vi "Autonomous Independent.vi"   [LabVIEW 2014]
doc: "This VI is called when autonomous begins, and will automatically be terminated when autonomous ends. You can carry out timed or sensor driven robot movement independently without needing to return to the caller."
uses:
  <vilib>/Rock Robotics/WPI/Relay/WPI_RelayValue.ctl
  <vilib>/Rock Robotics/Network Tables/SD Read String.vi
  <vilib>/Rock Robotics/WPI/RobotDrive/WPI_RobotDriveGetSetRefNum.vi
  Robot Global Data.vi
  <vilib>/Rock Robotics/WPI/RobotDrive/WPI_RobotDriveMecanumDrive_Cartesian.vi
  <vilib>/addons/control/pid/pid.llb/PID (DBL).vi
  <vilib>/Rock Robotics/Network Tables/SD Write Number.vi
  <vilib>/Rock Robotics/Network Tables/SD Write Numeric Array.vi
  SimpleGyro/SimpleGyro.lvlib
  <vilib>/addons/control/pid/NI_PID_pid.lvlib
panel:
  # "Be sure to right-click and choose Data Operations>>Make Current Value default if you want to save the array values with the VI"
types:
  T1 = typedef "WPI_RelayValue.ctl" = enum16{"Off", "On", "Forward", "Reverse"}
  T2 = cluster{"proportional gain (Kc)":dbl, "integral time (Ti, min)":dbl, "derivative time (Td, min)":dbl}
  T3 = typedef "SimpleGyro.lvlib/WPI_SimpleGyroDevRef.ctl" = cluster{"DevStatus":errorcluster, "Handle":i32, "Controller":T4, "SPI Bus":T5, "Device Found":bool, "Sample Rate":dbl}
  T4 = typedef "FPGA_TypedefDigitalModule.ctl" = enum16{"Controller 1"}
  T5 = typedef "spi_bus.ctl" = enum16{"SPI On-Board, CS0", "SPI On-Board, CS1", "SPI On-Board, CS2", "SPI On-Board, CS3", "SPI MXP", "Invalid"}
  T6 = typedef "WPI_RobotDriveDevRef.ctl" = cluster{"DevStatus":errorcluster, "Motors[]":T7[], "Square Inputs":bool, "Max Output":dbl}
  T7 = typedef "WPI_MotorControlDeviceRef.ctl" = cluster{"DeviceStatus":errorcluster, "Type":T8, "PWM":cluster{"Controller":T4, "PWM Channel":T9, "DeadBand":T10}, "CAN":cluster{"Device Number":u8, "Control Mode":T11, "Semaphore":T12, "Max Vout":dbl, "TalonSRX Control Mode":T13}, "Invert":bool, "TransformRef":T14, "InvTransformRef":T14}
  T8 = typedef "WPI_MotorControlType.ctl" = enum16{"PWM", "CAN", "CANTalonSRX"}
  T9 = typedef "FPGA_DIOPWMChannel.ctl" = enum8{"PWM 0", "PWM 1", "PWM 2", "PWM 3", "PWM 4", "PWM 5", "PWM 6", "PWM 7", "PWM 8", "PWM 9", "PWM MXP 0", "PWM MXP 1", "PWM MXP 2", "PWM MXP 3", "PWM MXP 4", "PWM MXP 5", "PWM MXP 6", "PWM MXP 7", "PWM MXP 8", "PWM MXP 9", "Invalid"}
  T10 = typedef "WPI_PWMDeadband.ctl" = cluster{"Name":string, "maxPositivePwm":i32, "minPositivePwm":i32, "centerPwm":i32, "maxNegativePwm":i32, "minNegativePwm":i32, "angularRange":u16}
  T11 = typedef "WPI_CANJaguar_ControlMode.ctl" = enum8{"Percent VBus", "Current", "Speed", "Position", "Voltage"}
  T12 = typedef "Semaphore RefNum" = refnum<k1>
  T13 = typedef "WPI_CANTalonSRX_APIControlMode.ctl" = enum8{"Percent VBus", "Speed", "Position", "Slave", "Unchanged / Invalid"}
  T14 = typedef "WPI_PWMTransform_ConPane.ctl" = refnum<vi>
  T15 = typedef "WPI_EncoderDevRef.ctl" = cluster{"DevStatus":errorcluster, "EncoderIndex":T16, "CounterIndex":T17, "DistancePerCount":dbl, "Decoding Type":T18}
  T16 = typedef "FPGA_EncoderIdx.ctl" = enum8{"Enc 0", "Enc 1", "Enc 2", "Enc 3", "Enc 4", "Enc 5", "Enc 6", "Enc 7", "Invalid"}
  T17 = typedef "FPGA_CounterCtrSystemIndex.ctl" = enum8{"Ctr 0", "Ctr 1", "Ctr 2", "Ctr 3", "Ctr 4", "Ctr 5", "Ctr 6", "Ctr 7", "Invalid"}
  T18 = typedef "WPI_EncoderType.ctl" = enum16{"1x", "2x", "4x"}
  T19 = typedef "WPI_RelayDevRef.ctl" = cluster{"DevStatus":errorcluster, "Relay Channel":T20, "Controller":T4, "Relay Direction":T21}
  T20 = typedef "FPGA_DIORelayChannel.ctl" = enum8{"Relay 0", "Relay 1", "Relay 2", "Relay 3", "Invalid"}
  T21 = typedef "WPI_RelayDirection.ctl" = enum16{"Both directions", "Forward only", "Reverse only"}
  T22 = cluster{"SimpleGyroDevRef":T3, "RobotDriveDevRef":T6, "EncoderDevRef":T15, "MotorControlDevRef":T7, "RelayDevRef":T19}
  T23 = cluster{"SimpleGyroDevRef":T3, "RobotDriveDevRef":T6, "EncoderDevRef":T15, "MotorControlDevRef":T7, "RelayDevRef":T19, "MotorControlDevRef":T7}
  T24 = cluster{"SimpleGyroDevRef":T3, "RobotDriveDevRef":T6, "EncoderDevRef":T15, "MotorControlDevRef":T7, "RelayDevRef":T19, "MotorControlDevRef":T7, "EncoderDevRef":T15}
  T25 = cluster{"SimpleGyroDevRef":T3, "RobotDriveDevRef":T6, "EncoderDevRef":T15, "MotorControlDevRef":T7, "RelayDevRef":T19, "MotorControlDevRef":T7, "EncoderDevRef":T15, "RelayDevRef":T19, "RelayDevRef":T19}
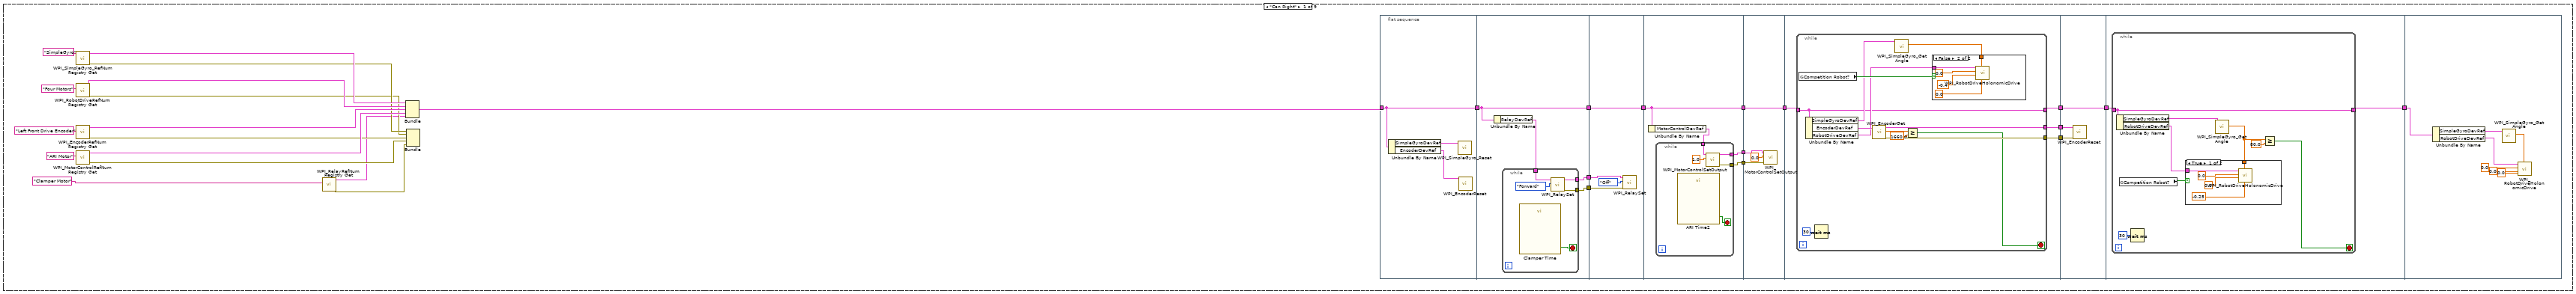
[diagram p2: hidden frame]
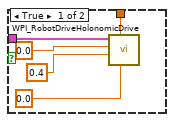
[diagram p3: hidden frame]
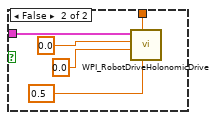
[diagram p4: hidden frame]
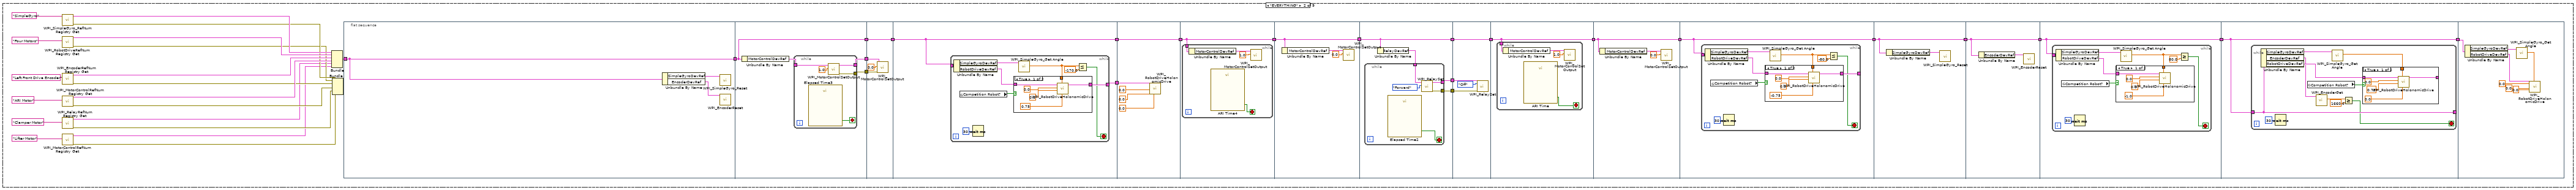
[diagram p5: hidden frame]
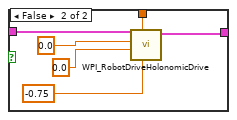
[diagram p6: hidden frame]
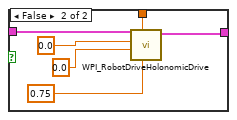
[diagram p7: hidden frame]
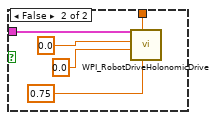
[diagram p8: hidden frame]
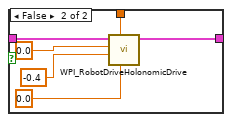
[diagram p9: hidden frame]
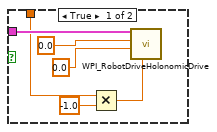
[diagram p11: hidden frame]
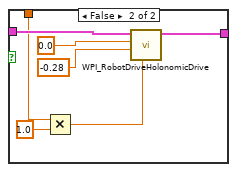
[diagram p12: hidden frame]
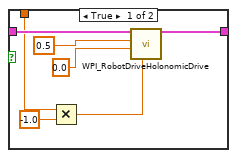
[diagram p13: hidden frame]
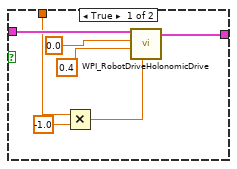
[diagram p14: hidden frame]
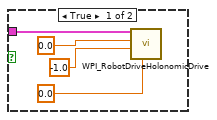
[diagram p15: hidden frame]
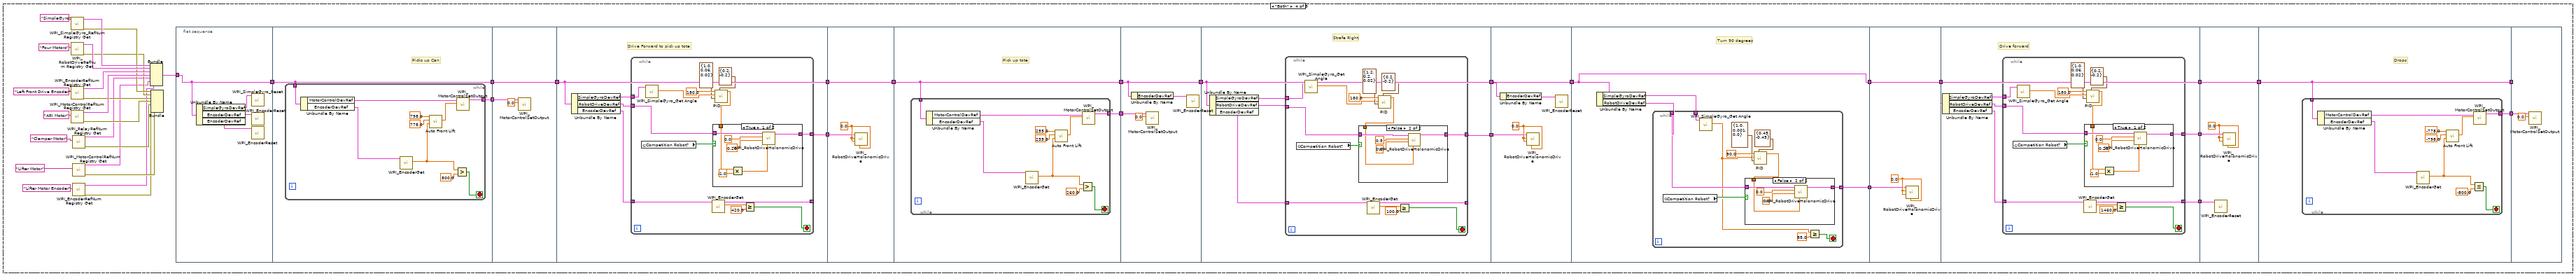
[diagram p16: hidden frame]
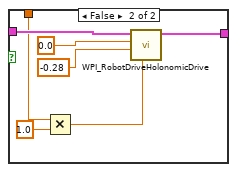
[diagram p17: hidden frame]
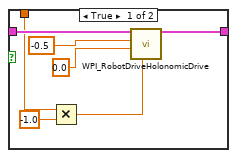
[diagram p18: hidden frame]
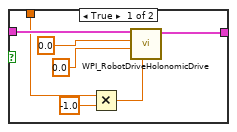
[diagram p19: hidden frame]
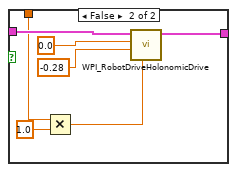
[diagram p20: hidden frame]
diagram:
  # "Every 20ms, report that we are running autonomous\ncode. Loop will abort the same time as the VI."
  n1 = call-poly <vilib>:"SD Read Value.vi"("Name"="AUTO") -> ("String"=w1:string)  [unwired: 8 in, 2 out]
  n2 = case shown="\"Dragon Tail\"" w1 {
    frame "Can Right" {
      n3 = call "WPI_SimpleGyro_RefNum Registry Get.vi"("refnum name"="SimpleGyro") -> ("error out"=w18:errorcluster, "SimpleGyroDevRef"=w22:T3)  [unwired: 9 in]
      n4 = call <vilib>:"WPI_RobotDriveRefNum Registry Get.vi"("refnum name"="Four Motors") -> ("error out"=w17:errorcluster, "RobotDriveDevRef"=w21:T6)  [unwired: 1 in, 8 out]
      n5 = call <vilib>:"WPI_EncoderRefNum Registry Get.vi"("refnum name"="Left Front Drive Encoder") -> ("error out"=w16:errorcluster, "EncoderDevRef"=w20:T15)  [unwired: 9 in]
      n6 = call <vilib>:"WPI_MotorControlRefNum Registry Get.vi"("refnum name"="ARI Motor") -> ("error out"=w15:errorcluster, "MotorControlDevRef"=w19:T7)  [unwired: 9 in]
      n7 = call <vilib>:"WPI_RelayRefNum Registry Get.vi"("refnum name"="Clamper Motor") -> ("error out"=w10:errorcluster, "RelayDevRef"=w11:T19)  [unwired: 9 in]
      n8 = Bundle("SimpleGyroDevRef"=w22, "RobotDriveDevRef"=w21, "EncoderDevRef"=w20, "MotorControlDevRef"=w19, "RelayDevRef"=w11) -> (w14:T22)  [unwired: 1 in]
      n9 = Bundle("error out"=w18, "error out"=w17, "error out"=w16, "error out"=w15, "error out"=w10) -> ()  [unwired: 1 in, 1 out]
      n10 = flat-sequence {
        tunnel: w14 -> [w33]
        tunnel: [w33] -> w13
        tunnel: [w39] -> w32
        tunnel: [w38] -> w31
        tunnel: w13 -> [w36]
        tunnel: [w36] -> w8
        tunnel: w32 -> [w47]
        tunnel: w31 -> [w46]
        tunnel: [w45] -> w9
        tunnel: w8 -> [w45]
        tunnel: [w52] -> w30
        tunnel: [w51] -> w29
        tunnel: w9 -> [w49]
        tunnel: [w49] -> w6
        tunnel: w30 -> [w60]
        tunnel: w29 -> [w59]
        tunnel: [w58] -> w7
        tunnel: w6 -> [w58]
        tunnel: [w65] -> w28
        tunnel: [w64] -> w27
        tunnel: w7 -> [w63]
        tunnel: [w62] -> w4
        tunnel: w28 -> [w90]
        tunnel: w27 -> [w89]
        tunnel: [w88] -> w5
        tunnel: w4 -> [w88]
        tunnel: w5 -> [w92]
        tunnel: [w91] -> w3
        tunnel: w3 -> [w113]
        frame #0 {
          n11 = Unbundle By Name(w33) -> ("SimpleGyroDevRef"=w35:T3, "EncoderDevRef"=w34:T15)
          n12 = call "WPI_SimpleGyro_Reset.vi"("SimpleGyroDevRef"=w35) -> ()  [unwired: 9 in, 2 out]
          n13 = call <vilib>:"WPI_EncoderReset.vi"("EncoderDevRef"=w34) -> ()  [unwired: 9 in, 2 out]
        }
        frame #1 {
          n14 = Unbundle By Name(w36) -> ("RelayDevRef"=w37:T19)
          n15 = while {
            tunnel: [w43] -> w39
            tunnel: [w42] -> w38
            tunnel: w37 -> [w40]
            stop <- w41 stop-if-true
            n16 = call "Clamper Time"() -> ("Time has Elapsed"=w41:bool)  [unwired: 12 in, 7 out]
            n17 = call <vilib>:"WPI_RelaySet.vi"("RelayValue"=WPI_RelayValue."Forward", "RelayDevRef"=w40) -> ("error out"=w42:errorcluster, "RelayDevRef"=w43:T19)  [unwired: 8 in]
          }
        }
        frame #2 {
          n18 = call <vilib>:"WPI_RelaySet.vi"("error in (no error)"=w46, "RelayValue"=WPI_RelayValue."Off", "RelayDevRef"=w47) -> ()  [unwired: 7 in, 2 out]
        }
        frame #3 {
          n19 = Unbundle By Name(w49) -> ("MotorControlDevRef"=w50:T7)
          n20 = while {
            tunnel: [w55] -> w52
            tunnel: [w54] -> w51
            tunnel: w50 -> [w53]
            stop <- w57 stop-if-true
            n21 = call "ARI Time2"() -> ("Time has Elapsed"=w57:bool)  [unwired: 12 in, 7 out]
            n22 = call <vilib>:"WPI_MotorControlSetOutput.vi"("Output"=1.0, "MotorControlDevRef"=w53) -> ("error out"=w55:errorcluster, "MotorControlDevRef"=w54:T7)  [unwired: 7 in, 1 out]
          }
        }
        frame #4 {
          n23 = call <vilib>:"WPI_MotorControlSetOutput.vi"("error in (no error)"=w60, "Output"=0.0, "MotorControlDevRef"=w59) -> ()  [unwired: 6 in, 3 out]
        }
        frame #5 {
          n24 = while {
            tunnel: [w75] -> w65
            tunnel: [w74] -> w64
            tunnel: w63 -> [w67]
            tunnel: [w67] -> w62
            stop <- w66 stop-if-true
            n25 = global read "Robot Global Data.vi" "Competition Robot?"() -> (w72:bool)
            n26 = Unbundle By Name(w67) -> ("SimpleGyroDevRef"=w70:T3, "EncoderDevRef"=w69:T15, "RobotDriveDevRef"=w68:T6)
            n27 = Wait (ms)(milliseconds to wait=u32 30) -> ()  [unwired: 1 out]
            n28 = call <vilib>:"WPI_EncoderGet.vi"("EncoderDevRef"=w69) -> ("error out"=w74:errorcluster, "Distance"=w77:dbl, "EncoderDevRef"=w75:T15)  [unwired: 5 in, 3 out]
            n29 = call "WPI_SimpleGyro_Get Angle.vi"("SimpleGyroDevRef"=w70) -> ("Angle"=w73:dbl)  [unwired: 8 in, 2 out]
            n30 = Greater Or Equal?(x=w77, y=1660.0) -> (x >= y?=w66:bool)
            n31 = case shown="False" w72 {
              tunnel: w73 -> [w79 w84]
              tunnel: w68 -> [w78 w83]
              frame True {
                n32 = call-poly <vilib>:"WPI_RobotDriveHolonomicDrive.vi"("Rotation"=0.0, "Gyro Angle"=w79, "Y"=0.4 ("X axis value"), "X"=0.0 ("X axis value"), "RobotDriveDevRef"=w78) -> ()  [unwired: 4 in, 3 out]
              }
              frame False {
                n33 = call-poly <vilib>:"WPI_RobotDriveHolonomicDrive.vi"("Rotation"=0.0, "Gyro Angle"=w84, "Y"=-0.4 ("X axis value"), "X"=0.0 ("X axis value"), "RobotDriveDevRef"=w83) -> ()  [unwired: 4 in, 3 out]
              }
            }
          }
        }
        frame #6 {
          n34 = call <vilib>:"WPI_EncoderReset.vi"("error in (no error)"=w89, "EncoderDevRef"=w90) -> ()  [unwired: 8 in, 2 out]
        }
        frame #7 {
          n35 = while {
            tunnel: w92 -> [w93]
            tunnel: [w93] -> w91
            stop <- w97 stop-if-true
            n36 = Unbundle By Name(w93) -> ("SimpleGyroDevRef"=w95:T3, "RobotDriveDevRef"=w94:T6)
            n37 = global read "Robot Global Data.vi" "Competition Robot?"() -> (w99:bool)
            n38 = Wait (ms)(milliseconds to wait=u32 30) -> ()  [unwired: 1 out]
            n39 = call "WPI_SimpleGyro_Get Angle.vi"("SimpleGyroDevRef"=w95) -> ("Angle"=w98:dbl)  [unwired: 8 in, 2 out]
            n40 = case shown="True" w99 {
              tunnel: w98 -> [w102 w107]
              tunnel: w94 -> [w101 w106]
              frame True {
                n41 = call-poly <vilib>:"WPI_RobotDriveHolonomicDrive.vi"("Rotation"=-0.25, "Gyro Angle"=w102, "Y"=0.0 ("X axis value"), "X"=0.0 ("X axis value"), "RobotDriveDevRef"=w101) -> ()  [unwired: 4 in, 3 out]
              }
              frame False {
                n42 = call-poly <vilib>:"WPI_RobotDriveHolonomicDrive.vi"("Rotation"=0.5, "Gyro Angle"=w107, "Y"=0.0 ("X axis value"), "X"=0.0 ("X axis value"), "RobotDriveDevRef"=w106) -> ()  [unwired: 4 in, 3 out]
              }
            }
            n43 = Greater Or Equal?(x=w98, y=80.0) -> (x >= y?=w97:bool)
          }
        }
        frame #8 {
          n44 = Unbundle By Name(w113) -> ("SimpleGyroDevRef"=w111:T3, "RobotDriveDevRef"=w112:T6)
          n45 = call "WPI_SimpleGyro_Get Angle.vi"("SimpleGyroDevRef"=w111) -> ("Angle"=w114:dbl)  [unwired: 8 in, 2 out]
          n46 = call-poly <vilib>:"WPI_RobotDriveHolonomicDrive.vi"("Rotation"=0.0, "Gyro Angle"=w114, "Y"=0.0, "X"=0.0, "RobotDriveDevRef"=w112) -> ()  [unwired: 4 in, 3 out]
        }
      }
    }
    frame "EVERYTHING" {
      n47 = call "WPI_SimpleGyro_RefNum Registry Get.vi"("refnum name"="SimpleGyro") -> ("error out"=w149:errorcluster, "SimpleGyroDevRef"=w153:T3)  [unwired: 9 in]
      n48 = call <vilib>:"WPI_RobotDriveRefNum Registry Get.vi"("refnum name"="Four Motors") -> ("error out"=w148:errorcluster, "RobotDriveDevRef"=w152:T6)  [unwired: 1 in, 8 out]
      n49 = call <vilib>:"WPI_EncoderRefNum Registry Get.vi"("refnum name"="Left Front Drive Encoder") -> ("error out"=w147:errorcluster, "EncoderDevRef"=w151:T15)  [unwired: 9 in]
      n50 = call <vilib>:"WPI_MotorControlRefNum Registry Get.vi"("refnum name"="ARI Motor") -> ("error out"=w146:errorcluster, "MotorControlDevRef"=w150:T7)  [unwired: 9 in]
      n51 = call <vilib>:"WPI_RelayRefNum Registry Get.vi"("refnum name"="Clamper Motor") -> ("error out"=w141:errorcluster, "RelayDevRef"=w142:T19)  [unwired: 9 in]
      n52 = call <vilib>:"WPI_MotorControlRefNum Registry Get.vi"("refnum name"="Lifter Motor") -> ("error out"=w118:errorcluster, "MotorControlDevRef"=w139:T7)  [unwired: 9 in]
      n53 = Bundle("SimpleGyroDevRef"=w153, "RobotDriveDevRef"=w152, "EncoderDevRef"=w151, "MotorControlDevRef"=w150, "RelayDevRef"=w142, "MotorControlDevRef"=w139) -> (w145:T23)  [unwired: 1 in]
      n54 = Bundle("error out"=w149, "error out"=w148, "error out"=w147, "error out"=w146, "error out"=w141, "error out"=w118) -> ()  [unwired: 1 in, 1 out]
      n55 = flat-sequence {
        tunnel: w145 -> [w158]
        tunnel: [w158] -> w144
        tunnel: w144 -> [w163]
        tunnel: [w163] -> w138
        tunnel: [w162] -> w136
        tunnel: [w161] -> w135
        tunnel: w138 -> [w173]
        tunnel: [w173] -> w137
        tunnel: w136 -> [w172]
        tunnel: w135 -> [w171]
        tunnel: w137 -> [w175]
        tunnel: [w175] -> w134
        tunnel: [w174] -> w133
        tunnel: w134 -> [w201]
        tunnel: [w201] -> w127
        tunnel: w133 -> [w200]
        tunnel: w127 -> [w202]
        tunnel: [w202] -> w126
        tunnel: w126 -> [w207]
        tunnel: [w207] -> w125
        tunnel: w125 -> [w212]
        tunnel: [w212] -> w132
        tunnel: [w211] -> w131
        tunnel: [w210] -> w130
        tunnel: w132 -> [w222]
        tunnel: [w222] -> w129
        tunnel: w131 -> [w220]
        tunnel: w130 -> [w219]
        tunnel: w129 -> [w223]
        tunnel: [w223] -> w128
        tunnel: w128 -> [w228]
        tunnel: [w228] -> w124
        tunnel: w124 -> [w231]
        tunnel: [w231] -> w123
        tunnel: w123 -> [w254]
        tunnel: [w254] -> w122
        tunnel: w122 -> [w256]
        tunnel: [w256] -> w121
        tunnel: w121 -> [w257]
        tunnel: [w257] -> w120
        tunnel: w120 -> [w276]
        tunnel: [w276] -> w119
        tunnel: w119 -> [w299]
        frame #0 {
          n56 = Unbundle By Name(w158) -> ("SimpleGyroDevRef"=w160:T3, "EncoderDevRef"=w159:T15)
          n57 = call "WPI_SimpleGyro_Reset.vi"("SimpleGyroDevRef"=w160) -> ()  [unwired: 9 in, 2 out]
          n58 = call <vilib>:"WPI_EncoderReset.vi"("EncoderDevRef"=w159) -> ()  [unwired: 9 in, 2 out]
        }
        frame #1 {
          n59 = Unbundle By Name(w163) -> ("MotorControlDevRef"=w164:T7)
          n60 = while {
            tunnel: w164 -> [w168]
            tunnel: [w166] -> w162
            tunnel: [w165] -> w161
            stop <- w169 stop-if-true
            n61 = call "Elapsed Time3"() -> ("Time has Elapsed"=w169:bool)  [unwired: 12 in, 7 out]
            n62 = call <vilib>:"WPI_MotorControlSetOutput.vi"("Output"=1.0, "MotorControlDevRef"=w168) -> ("error out"=w165:errorcluster, "MotorControlDevRef"=w166:T7)  [unwired: 7 in, 1 out]
          }
        }
        frame #2 {
          n63 = call <vilib>:"WPI_MotorControlSetOutput.vi"("error in (no error)"=w171, "Output"=0.0, "MotorControlDevRef"=w172) -> ()  [unwired: 6 in, 3 out]
        }
        frame #3 {
          n64 = while {
            tunnel: w175 -> [w179]
            tunnel: [w177] -> w174
            stop <- w176 stop-if-true
            n65 = Unbundle By Name(w179) -> ("SimpleGyroDevRef"=w178:T3, "RobotDriveDevRef"=w180:T6)
            n66 = global read "Robot Global Data.vi" "Competition Robot?"() -> (w183:bool)
            n67 = Wait (ms)(milliseconds to wait=u32 30) -> ()  [unwired: 1 out]
            n68 = call "WPI_SimpleGyro_Get Angle.vi"("SimpleGyroDevRef"=w178) -> ("Angle"=w182:dbl)  [unwired: 8 in, 2 out]
            n69 = case shown="True" w183 {
              tunnel: w182 -> [w187 w193]
              tunnel: w180 -> [w186 w191]
              tunnel: [w185 w192] -> w177
              frame True {
                n70 = call-poly <vilib>:"WPI_RobotDriveHolonomicDrive.vi"("Rotation"=0.75, "Gyro Angle"=w187, "Y"=0.0 ("X axis value"), "X"=0.0 ("X axis value"), "RobotDriveDevRef"=w186) -> ("RobotDriveDevRef"=w185:T6)  [unwired: 4 in, 2 out]
              }
              frame False {
                n71 = call-poly <vilib>:"WPI_RobotDriveHolonomicDrive.vi"("Rotation"=-0.75, "Gyro Angle"=w193, "Y"=0.0 ("X axis value"), "X"=0.0 ("X axis value"), "RobotDriveDevRef"=w191) -> ("RobotDriveDevRef"=w192:T6)  [unwired: 4 in, 2 out]
              }
            }
            n72 = Less Or Equal?(x=w182, y=-170.0) -> (x <= y?=w176:bool)
          }
        }
        frame #4 {
          n73 = call-poly <vilib>:"WPI_RobotDriveHolonomicDrive.vi"("Rotation"=0.0, "Y"=0.0, "X"=0.0, "RobotDriveDevRef"=w200) -> ()  [unwired: 5 in, 3 out]
        }
        frame #5 {
          n74 = while {
            tunnel: w202 -> [w203]
            stop <- w206 stop-if-true
            n75 = Unbundle By Name(w203) -> ("MotorControlDevRef"=w205:T7)
            n76 = call "ARI Time4"() -> ("Time has Elapsed"=w206:bool)  [unwired: 12 in, 7 out]
            n77 = call <vilib>:"WPI_MotorControlSetOutput.vi"("Output"=1.0, "MotorControlDevRef"=w205) -> ()  [unwired: 7 in, 3 out]
          }
        }
        frame #6 {
          n78 = Unbundle By Name(w207) -> ("MotorControlDevRef"=w208:T7)
          n79 = call <vilib>:"WPI_MotorControlSetOutput.vi"("Output"=0.0, "MotorControlDevRef"=w208) -> ()  [unwired: 7 in, 3 out]
        }
        frame #7 {
          n80 = Unbundle By Name(w212) -> ("RelayDevRef"=w213:T19)
          n81 = while {
            tunnel: [w217] -> w211
            tunnel: [w216] -> w210
            tunnel: w213 -> [w214]
            stop <- w215 stop-if-true
            n82 = call "Elapsed Time2"() -> ("Time has Elapsed"=w215:bool)  [unwired: 12 in, 7 out]
            n83 = call <vilib>:"WPI_RelaySet.vi"("RelayValue"=WPI_RelayValue."Forward", "RelayDevRef"=w214) -> ("error out"=w216:errorcluster, "RelayDevRef"=w217:T19)  [unwired: 8 in]
          }
        }
        frame #8 {
          n84 = call <vilib>:"WPI_RelaySet.vi"("error in (no error)"=w219, "RelayValue"=WPI_RelayValue."Off", "RelayDevRef"=w220) -> ()  [unwired: 7 in, 2 out]
        }
        frame #9 {
          n85 = while {
            tunnel: w223 -> [w224]
            stop <- w227 stop-if-true
            n86 = Unbundle By Name(w224) -> ("MotorControlDevRef"=w226:T7)
            n87 = call "ARI Time"() -> ("Time has Elapsed"=w227:bool)  [unwired: 12 in, 7 out]
            n88 = call <vilib>:"WPI_MotorControlSetOutput.vi"("Output"=1.0, "MotorControlDevRef"=w226) -> ()  [unwired: 7 in, 3 out]
          }
        }
        frame #10 {
          n89 = Unbundle By Name(w228) -> ("MotorControlDevRef"=w229:T7)
          n90 = call <vilib>:"WPI_MotorControlSetOutput.vi"("Output"=0.0, "MotorControlDevRef"=w229) -> ()  [unwired: 7 in, 3 out]
        }
        frame #11 {
          n91 = while {
            tunnel: w231 -> [w235]
            tunnel: [w233] -> _
            stop <- w232 stop-if-true
            n92 = Unbundle By Name(w235) -> ("SimpleGyroDevRef"=w234:T3, "RobotDriveDevRef"=w236:T6)
            n93 = global read "Robot Global Data.vi" "Competition Robot?"() -> (w239:bool)
            n94 = Wait (ms)(milliseconds to wait=u32 30) -> ()  [unwired: 1 out]
            n95 = call "WPI_SimpleGyro_Get Angle.vi"("SimpleGyroDevRef"=w234) -> ("Angle"=w238:dbl)  [unwired: 8 in, 2 out]
            n96 = case shown="True" w239 {
              tunnel: w238 -> [w243 w249]
              tunnel: w236 -> [w242 w247]
              tunnel: [w241 w248] -> w233
              frame True {
                n97 = call-poly <vilib>:"WPI_RobotDriveHolonomicDrive.vi"("Rotation"=-0.75, "Gyro Angle"=w243, "Y"=0.0 ("X axis value"), "X"=0.0 ("X axis value"), "RobotDriveDevRef"=w242) -> ("RobotDriveDevRef"=w241:T6)  [unwired: 4 in, 2 out]
              }
              frame False {
                n98 = call-poly <vilib>:"WPI_RobotDriveHolonomicDrive.vi"("Rotation"=0.75, "Gyro Angle"=w249, "Y"=0.0 ("X axis value"), "X"=0.0 ("X axis value"), "RobotDriveDevRef"=w247) -> ("RobotDriveDevRef"=w248:T6)  [unwired: 4 in, 2 out]
              }
            }
            n99 = Less Or Equal?(x=w238, y=-80.0) -> (x <= y?=w232:bool)
          }
        }
        frame #12 {
          n100 = Unbundle By Name(w254) -> ("SimpleGyroDevRef"=w253:T3)
          n101 = call "WPI_SimpleGyro_Reset.vi"("SimpleGyroDevRef"=w253) -> ()  [unwired: 9 in, 2 out]
        }
        frame #13 {
          n102 = Unbundle By Name(w256) -> ("EncoderDevRef"=w255:T15)
          n103 = call <vilib>:"WPI_EncoderReset.vi"("EncoderDevRef"=w255) -> ()  [unwired: 9 in, 2 out]
        }
        frame #14 {
          n104 = while {
            tunnel: w257 -> [w259]
            stop <- w260 stop-if-true
            n105 = Unbundle By Name(w259) -> ("SimpleGyroDevRef"=w258:T3, "RobotDriveDevRef"=w261:T6)
            n106 = global read "Robot Global Data.vi" "Competition Robot?"() -> (w264:bool)
            n107 = Wait (ms)(milliseconds to wait=u32 30) -> ()  [unwired: 1 out]
            n108 = call "WPI_SimpleGyro_Get Angle.vi"("SimpleGyroDevRef"=w258) -> ("Angle"=w263:dbl)  [unwired: 8 in, 2 out]
            n109 = case shown="True" w264 {
              tunnel: w263 -> [w267 w272]
              tunnel: w261 -> [w266 w271]
              frame True {
                n110 = call-poly <vilib>:"WPI_RobotDriveHolonomicDrive.vi"("Rotation"=-1.0, "Gyro Angle"=w267, "Y"=0.0 ("X axis value"), "X"=0.0 ("X axis value"), "RobotDriveDevRef"=w266) -> ()  [unwired: 4 in, 3 out]
              }
              frame False {
                n111 = call-poly <vilib>:"WPI_RobotDriveHolonomicDrive.vi"("Rotation"=0.75, "Gyro Angle"=w272, "Y"=0.0 ("X axis value"), "X"=0.0 ("X axis value"), "RobotDriveDevRef"=w271) -> ()  [unwired: 4 in, 3 out]
              }
            }
            n112 = Greater Or Equal?(x=w263, y=80.0) -> (x >= y?=w260:bool)
          }
        }
        frame #15 {
          n113 = while {
            tunnel: w276 -> [w281]
            tunnel: [w281] -> _
            stop <- w280 stop-if-true
            n114 = Unbundle By Name(w281) -> ("SimpleGyroDevRef"=w278:T3, "EncoderDevRef"=w277:T15, "RobotDriveDevRef"=w279:T6)
            n115 = Wait (ms)(milliseconds to wait=u32 30) -> ()  [unwired: 1 out]
            n116 = global read "Robot Global Data.vi" "Competition Robot?"() -> (w283:bool)
            n117 = call <vilib>:"WPI_EncoderGet.vi"("EncoderDevRef"=w277) -> ("Distance"=w286:dbl)  [unwired: 5 in, 5 out]
            n118 = call "WPI_SimpleGyro_Get Angle.vi"("SimpleGyroDevRef"=w278) -> ("Angle"=w284:dbl)  [unwired: 8 in, 2 out]
            n119 = Greater Or Equal?(x=w286, y=1660.0) -> (x >= y?=w280:bool)
            n120 = case shown="True" w283 {
              tunnel: w284 -> [w289 w295]
              tunnel: w279 -> [w287 w294]
              tunnel: [w288 w293] -> _
              frame True {
                n121 = call-poly <vilib>:"WPI_RobotDriveHolonomicDrive.vi"("Rotation"=0.0, "Gyro Angle"=w289, "Y"=0.75 ("X axis value"), "X"=0.0 ("X axis value"), "RobotDriveDevRef"=w287) -> ("RobotDriveDevRef"=w288:T6)  [unwired: 4 in, 2 out]
              }
              frame False {
                n122 = call-poly <vilib>:"WPI_RobotDriveHolonomicDrive.vi"("Rotation"=0.0, "Gyro Angle"=w295, "Y"=-0.4 ("X axis value"), "X"=0.0 ("X axis value"), "RobotDriveDevRef"=w294) -> ("RobotDriveDevRef"=w293:T6)  [unwired: 4 in, 2 out]
              }
            }
          }
        }
        frame #16 {
          n123 = Unbundle By Name(w299) -> ("SimpleGyroDevRef"=w300:T3, "RobotDriveDevRef"=w301:T6)
          n124 = call "WPI_SimpleGyro_Get Angle.vi"("SimpleGyroDevRef"=w300) -> ("Angle"=w302:dbl)  [unwired: 8 in, 2 out]
          n125 = call-poly <vilib>:"WPI_RobotDriveHolonomicDrive.vi"("Rotation"=0.0, "Gyro Angle"=w302, "Y"=0.0, "X"=0.0, "RobotDriveDevRef"=w301) -> ()  [unwired: 4 in, 3 out]
        }
      }
    }
    frame "Totes Totes" {
      n126 = call "WPI_SimpleGyro_RefNum Registry Get.vi"("refnum name"="SimpleGyro") -> ("error out"=w347:errorcluster, "SimpleGyroDevRef"=w351:T3)  [unwired: 9 in]
      n127 = call <vilib>:"WPI_RobotDriveRefNum Registry Get.vi"("refnum name"="Four Motors") -> ("error out"=w346:errorcluster, "RobotDriveDevRef"=w350:T6)  [unwired: 1 in, 8 out]
      n128 = call <vilib>:"WPI_EncoderRefNum Registry Get.vi"("refnum name"="Left Front Drive Encoder") -> ("error out"=w345:errorcluster, "EncoderDevRef"=w349:T15)  [unwired: 9 in]
      n129 = call <vilib>:"WPI_MotorControlRefNum Registry Get.vi"("refnum name"="ARI Motor") -> ("error out"=w344:errorcluster, "MotorControlDevRef"=w348:T7)  [unwired: 9 in]
      n130 = call <vilib>:"WPI_RelayRefNum Registry Get.vi"("refnum name"="Clamper Motor") -> ("error out"=w341:errorcluster, "RelayDevRef"=w342:T19)  [unwired: 9 in]
      n131 = call <vilib>:"WPI_MotorControlRefNum Registry Get.vi"("refnum name"="Lifter Motor") -> ("error out"=w337:errorcluster, "MotorControlDevRef"=w338:T7)  [unwired: 9 in]
      n132 = call <vilib>:"WPI_EncoderRefNum Registry Get.vi"("refnum name"="Lifter Motor Encoder") -> ("error out"=w307:errorcluster, "EncoderDevRef"=w308:T15)  [unwired: 9 in]
      n133 = Bundle("SimpleGyroDevRef"=w351, "RobotDriveDevRef"=w350, "EncoderDevRef"=w349, "MotorControlDevRef"=w348, "RelayDevRef"=w342, "MotorControlDevRef"=w338, "EncoderDevRef"=w308) -> (w314:T24)  [unwired: 1 in]
      n134 = Bundle("error out"=w347, "error out"=w346, "error out"=w345, "error out"=w344, "error out"=w341, "error out"=w337, "error out"=w307) -> ()  [unwired: 1 in, 1 out]
      n135 = flat-sequence {
        tunnel: w314 -> [w357]
        tunnel: [w357] -> w340
        tunnel: w340 -> [w362]
        tunnel: [w362] -> w336
        tunnel: [w361] -> w335
        tunnel: [w360] -> w334
        tunnel: w336 -> [w390]
        tunnel: w335 -> [w394]
        tunnel: w334 -> [w392]
        tunnel: [w390] -> w306
        tunnel: [w395] -> w319
        tunnel: w306 -> [w395]
        tunnel: w319 -> [w419]
        tunnel: [w419] -> w318
        tunnel: w318 -> [w423]
        tunnel: [w423] -> w321
        tunnel: [w422] -> w320
        tunnel: [w420] -> w313
        tunnel: w321 -> [w457]
        tunnel: [w457] -> w316
        tunnel: w320 -> [w456]
        tunnel: w313 -> [w455]
        tunnel: w316 -> [w458]
        tunnel: [w458] -> w315
        tunnel: w315 -> [w463]
        tunnel: [w463] -> w333
        tunnel: [w461] -> w332
        tunnel: w333 -> [w473]
        tunnel: w332 -> [w475]
        tunnel: [w473] -> w317
        tunnel: w317 -> [w479]
        tunnel: [w479] -> w331
        tunnel: [w478] -> w330
        tunnel: [w476] -> w312
        tunnel: w331 -> [w511]
        tunnel: w330 -> [w510]
        tunnel: [w511] -> w329
        tunnel: w312 -> [w509]
        tunnel: w329 -> [w514]
        tunnel: [w514] -> w328
        tunnel: [w515] -> w327
        tunnel: [w512] -> w311
        tunnel: w328 -> [w545]
        tunnel: w327 -> [w547]
        tunnel: w311 -> [w546]
        tunnel: [w545] -> w310
        tunnel: w310 -> [w548]
        tunnel: [w548] -> w326
        tunnel: w326 -> [w569]
        tunnel: [w569] -> w325
        tunnel: [w568] -> w324
        tunnel: [w567] -> w323
        tunnel: w325 -> [w600]
        tunnel: w324 -> [w599]
        tunnel: w323 -> [w598]
        tunnel: [w600] -> w322
        tunnel: [w601] -> _
        tunnel: w322 -> [w601]
        frame #0 {
          n136 = Unbundle By Name(w357) -> ("SimpleGyroDevRef"=w358:T3, "EncoderDevRef"=w359:T15, "EncoderDevRef"=w356:T15)
          n137 = call "WPI_SimpleGyro_Reset.vi"("SimpleGyroDevRef"=w358) -> ()  [unwired: 9 in, 2 out]
          n138 = call <vilib>:"WPI_EncoderReset.vi"("EncoderDevRef"=w359) -> ()  [unwired: 9 in, 2 out]
          n139 = call <vilib>:"WPI_EncoderReset.vi"("EncoderDevRef"=w356) -> ()  [unwired: 9 in, 2 out]
        }
        frame #1 {
          # "Simultaneously lowers ARI"
          # "Picks up tote"
          n140 = while {
            tunnel: w362 -> [w373]
            tunnel: [w365] -> w361
            tunnel: [w364] -> w360
            stop <- w370 stop-if-true
            n141 = Unbundle By Name(w373) -> ("MotorControlDevRef"=w372:T7, "MotorControlDevRef"=w371:T7, "EncoderDevRef"=w363:T15)
            n142 = while {
              tunnel: w372 -> [w389]
              tunnel: [w387] -> w368
              tunnel: [w388] -> w365
              tunnel: w363 -> [w385]
              stop <- w387 stop-if-true
              n143 = call <vilib>:"WPI_EncoderGet.vi"("EncoderDevRef"=w385) -> ("Distance"=w384:dbl)  [unwired: 5 in, 5 out]
              n144 = call "Auto Front Lift.vi"("Encoder Input"=w384, "Lower Range"=315.0 ("y"), "Upper Range"=335.0 ("y")) -> ("Output"=w383:dbl)  [unwired: 8 in]
              n145 = Greater?(x=w384, y=250.0) -> (0:w387:bool)
              n146 = call <vilib>:"WPI_MotorControlSetOutput.vi"("Output"=w383, "MotorControlDevRef"=w389) -> ("MotorControlDevRef"=w388:T7)  [unwired: 7 in, 2 out]
            }
            n147 = global read "Robot Global Data.vi" "Competition Robot?"() -> (w369:bool)
            n148 = while {
              tunnel: w371 -> [w380]
              tunnel: w369 -> [w378]
              tunnel: [w375] -> w367
              tunnel: [w374] -> w364
              stop <- w375 stop-if-true
              n149 = Select(t=-1.0, s=w378, f=0.0) -> (s? t:f=w379:dbl)
              n150 = call "ARI Time5"() -> ("Time has Elapsed"=w375:bool)  [unwired: 12 in, 7 out]
              n151 = call <vilib>:"WPI_MotorControlSetOutput.vi"("Output"=w379, "MotorControlDevRef"=w380) -> ("MotorControlDevRef"=w374:T7)  [unwired: 7 in, 2 out]
            }
            n152 = And(x=w367, y=w368) -> (x .and. y?=w366:bool)
            n153 = Select(t=w366, s=w369, f=w368) -> (s? t:f=w370:bool)
          }
        }
        frame #2 {
          n154 = call <vilib>:"WPI_MotorControlSetOutput.vi"("Output"=0.0, "MotorControlDevRef"=w394) -> ()  [unwired: 7 in, 3 out]
          n155 = call <vilib>:"WPI_MotorControlSetOutput.vi"("Output"=0.0, "MotorControlDevRef"=w392) -> ()  [unwired: 7 in, 3 out]
        }
        frame #3 {
          # "Turns 180 degrees while carrying tote"
          n156 = Unbundle By Name(w395) -> ("SimpleGyroDevRef"=w397:T3, "RobotDriveDevRef"=w396:T6)
          n157 = while {
            tunnel: w397 -> [w404]
            tunnel: w396 -> [w403]
            stop <- w405 stop-if-true
            n158 = global read "Robot Global Data.vi" "Competition Robot?"() -> (w406:bool)
            n159 = call "WPI_SimpleGyro_Get Angle.vi"("SimpleGyroDevRef"=w404) -> ("Angle"=w398:dbl)  [unwired: 8 in, 2 out]
            n160 = call-poly <vilib>:"PID.vi"("output range"=cluster{"output high":dbl, "output low":dbl} {"output high"=0.45, "output low"=-0.45}, "PID gains"=T2 {"proportional gain (Kc)"=1.0, "integral time (Ti, min)"=0.001, "derivative time (Td, min)"=0.0}, "process variable"=w398, "setpoint"=180.0) -> ("output"=w399:dbl)  [unwired: 6 in, 1 out]
            n161 = case shown="False" w406 {
              tunnel: w403 -> [w411 w415]
              tunnel: w399 -> [w410 w414]
              frame True {
                n162 = Multiply(x=w410, y=-1.0) -> (x*y=w408:dbl)
                n163 = call-poly <vilib>:"WPI_RobotDriveHolonomicDrive.vi"("Rotation"=w408, "Y"=0.0 ("X axis value"), "X"=0.0 ("X axis value"), "RobotDriveDevRef"=w411) -> ()  [unwired: 5 in, 3 out]
              }
              frame False {
                n164 = call-poly <vilib>:"WPI_RobotDriveHolonomicDrive.vi"("Rotation"=w414, "Y"=0.0 ("X axis value"), "X"=0.0 ("X axis value"), "RobotDriveDevRef"=w415) -> ()  [unwired: 5 in, 3 out]
              }
            }
            n165 = Greater Or Equal?(x=w398, y=172.0) -> (x >= y?=w405:bool)
          }
        }
        frame #4 {
          n166 = Unbundle By Name(w419) -> ("EncoderDevRef"=w418:T15)
          n167 = call <vilib>:"WPI_EncoderReset.vi"("EncoderDevRef"=w418) -> ()  [unwired: 9 in, 2 out]
        }
        frame #5 {
          # "Drive Forward to pick up tote #2"
          n168 = Unbundle By Name(w423) -> ("SimpleGyroDevRef"=w421:T3, "RobotDriveDevRef"=w425:T6, "EncoderDevRef"=w424:T15)
          n169 = while {
            tunnel: w425 -> [w435]
            tunnel: w424 -> [w434]
            tunnel: [w433] -> w422
            tunnel: w421 -> [w430]
            tunnel: [w426] -> w420
            stop <- w436 stop-if-true
            n170 = global read "Robot Global Data.vi" "Competition Robot?"() -> (w439:bool)
            n171 = call "WPI_SimpleGyro_Get Angle.vi"("SimpleGyroDevRef"=w430) -> ("Angle"=w429:dbl)  [unwired: 8 in, 2 out]
            n172 = call <vilib>:"WPI_EncoderGet.vi"("EncoderDevRef"=w434) -> ("Distance"=w438:dbl, "EncoderDevRef"=w433:T15)  [unwired: 5 in, 4 out]
            n173 = call-poly <vilib>:"PID.vi"("output range"=cluster{"output high":dbl, "output low":dbl} {"output high"=0.2, "output low"=-0.2}, "PID gains"=T2 {"proportional gain (Kc)"=1.0, "integral time (Ti, min)"=0.06, "derivative time (Td, min)"=0.02}, "process variable"=w429, "setpoint"=180.0) -> ("output"=w427:dbl)  [unwired: 6 in, 1 out]
            n174 = case shown="True" w439 {
              tunnel: w435 -> [w444 w451]
              tunnel: w427 -> [w442 w450]
              tunnel: [w441 w448] -> w426
              frame True {
                n175 = Multiply(x=w442, y=-1.0) -> (x*y=w440:dbl)
                n176 = call-poly <vilib>:"WPI_RobotDriveHolonomicDrive.vi"("Rotation"=w440, "Y"=0.28 ("X axis value"), "X"=0.0 ("X axis value"), "RobotDriveDevRef"=w444) -> ("RobotDriveDevRef"=w441:T6)  [unwired: 5 in, 2 out]
              }
              frame False {
                n177 = Multiply(x=w450, y=1.0) -> (x*y=w447:dbl)
                n178 = call-poly <vilib>:"WPI_RobotDriveHolonomicDrive.vi"("Rotation"=w447, "Y"=-0.28 ("X axis value"), "X"=0.0 ("X axis value"), "RobotDriveDevRef"=w451) -> ("RobotDriveDevRef"=w448:T6)  [unwired: 5 in, 2 out]
              }
            }
            n179 = Greater Or Equal?(x=w438, y=420.0) -> (x >= y?=w436:bool)
          }
        }
        frame #6 {
          w454 = 0.0 ("X")
          n180 = call <vilib>:"WPI_EncoderReset.vi"("EncoderDevRef"=w456) -> ()  [unwired: 9 in, 2 out]
          n181 = call-poly <vilib>:"WPI_RobotDriveHolonomicDrive.vi"("Rotation"=w454, "Y"=w454, "X"=w454, "RobotDriveDevRef"=w455) -> ()  [unwired: 5 in, 3 out]
        }
        frame #7 {
          n182 = while {
            stop <- w459 stop-if-true
            n183 = call "Elapsed Time9"() -> ("Time has Elapsed"=w459:bool)  [unwired: 12 in, 7 out]
          }
        }
        frame #8 {
          # "Picks up second tote"
          n184 = Unbundle By Name(w463) -> ("MotorControlDevRef"=w462:T7, "EncoderDevRef"=w460:T15)
          n185 = while {
            tunnel: w462 -> [w472]
            tunnel: [w471] -> w461
            tunnel: w460 -> [w468]
            stop <- w470 stop-if-true
            n186 = call <vilib>:"WPI_EncoderGet.vi"("EncoderDevRef"=w468) -> ("Distance"=w464:dbl)  [unwired: 5 in, 5 out]
            n187 = call "Auto Front Lift.vi"("Encoder Input"=w464, "Lower Range"=625.0 ("y"), "Upper Range"=645.0 ("y")) -> ("Output"=w465:dbl)  [unwired: 8 in]
            n188 = call <vilib>:"WPI_MotorControlSetOutput.vi"("Output"=w465, "MotorControlDevRef"=w472) -> ("MotorControlDevRef"=w471:T7)  [unwired: 7 in, 2 out]
            n189 = Greater?(x=w464, y=500.0) -> (0:w470:bool)
          }
        }
        frame #9 {
          n190 = call <vilib>:"WPI_MotorControlSetOutput.vi"("Output"=0.0, "MotorControlDevRef"=w475) -> ()  [unwired: 7 in, 3 out]
        }
        frame #10 {
          # "Strafe Left Around Tote #2"
          n191 = Unbundle By Name(w479) -> ("SimpleGyroDevRef"=w477:T3, "RobotDriveDevRef"=w481:T6, "EncoderDevRef"=w480:T15)
          n192 = while {
            tunnel: w481 -> [w491]
            tunnel: w480 -> [w490]
            tunnel: [w489] -> w478
            tunnel: w477 -> [w485]
            tunnel: [w482] -> w476
            stop <- w492 stop-if-true
            n193 = global read "Robot Global Data.vi" "Competition Robot?"() -> (w495:bool)
            n194 = call "WPI_SimpleGyro_Get Angle.vi"("SimpleGyroDevRef"=w485) -> ("Angle"=w484:dbl)  [unwired: 8 in, 2 out]
            n195 = call <vilib>:"WPI_EncoderGet.vi"("EncoderDevRef"=w490) -> ("Distance"=w494:dbl, "EncoderDevRef"=w489:T15)  [unwired: 5 in, 4 out]
            n196 = call-poly <vilib>:"PID.vi"("output range"=cluster{"output high":dbl, "output low":dbl} {"output high"=0.2, "output low"=-0.2}, "PID gains"=T2 {"proportional gain (Kc)"=1.2, "integral time (Ti, min)"=0.2, "derivative time (Td, min)"=0.02}, "process variable"=w484, "setpoint"=180.0) -> ("output"=w483:dbl)  [unwired: 6 in, 1 out]
            n197 = case shown="False" w495 {
              tunnel: w491 -> [w500 w505]
              tunnel: w483 -> [w499 w503]
              tunnel: [w497 w504] -> w482
              frame True {
                n198 = Multiply(x=w499, y=-1.0) -> (x*y=w496:dbl)
                n199 = call-poly <vilib>:"WPI_RobotDriveHolonomicDrive.vi"("Rotation"=w496, "Y"=0.0 ("X axis value"), "X"=0.5 ("X axis value"), "RobotDriveDevRef"=w500) -> ("RobotDriveDevRef"=w497:T6)  [unwired: 5 in, 2 out]
              }
              frame False {
                n200 = call-poly <vilib>:"WPI_RobotDriveHolonomicDrive.vi"("Rotation"=w503, "Y"=0.0 ("X axis value"), "X"=-0.5 ("X axis value"), "RobotDriveDevRef"=w505) -> ("RobotDriveDevRef"=w504:T6)  [unwired: 5 in, 2 out]
              }
            }
            n201 = Less Or Equal?(x=w494, y=-560.0) -> (x <= y?=w492:bool)
          }
        }
        frame #11 {
          w508 = 0.0 ("X")
          # "Stop Motors"
          n202 = call <vilib>:"WPI_EncoderReset.vi"("EncoderDevRef"=w510) -> ()  [unwired: 9 in, 2 out]
          n203 = call-poly <vilib>:"WPI_RobotDriveHolonomicDrive.vi"("Rotation"=w508, "Y"=w508, "X"=w508, "RobotDriveDevRef"=w509) -> ()  [unwired: 5 in, 3 out]
        }
        frame #12 {
          # "Drive Forward to Tote #3"
          n204 = Unbundle By Name(w514) -> ("SimpleGyroDevRef"=w513:T3, "RobotDriveDevRef"=w517:T6, "EncoderDevRef"=w516:T15)
          n205 = while {
            tunnel: w517 -> [w527]
            tunnel: w516 -> [w526]
            tunnel: [w525] -> w515
            tunnel: w513 -> [w520]
            tunnel: [w518] -> w512
            stop <- w528 stop-if-true
            n206 = global read "Robot Global Data.vi" "Competition Robot?"() -> (w531:bool)
            n207 = call "WPI_SimpleGyro_Get Angle.vi"("SimpleGyroDevRef"=w520) -> ("Angle"=w521:dbl)  [unwired: 8 in, 2 out]
            n208 = call-poly <vilib>:"PID.vi"("output range"=cluster{"output high":dbl, "output low":dbl} {"output high"=0.19, "output low"=-0.2}, "PID gains"=T2 {"proportional gain (Kc)"=1.0, "integral time (Ti, min)"=0.3, "derivative time (Td, min)"=0.01}, "process variable"=w521, "setpoint"=180.0) -> ("output"=w519:dbl)  [unwired: 6 in, 1 out]
            n209 = case shown="False" w531 {
              tunnel: w527 -> [w536 w541]
              tunnel: w519 -> [w535 w539]
              tunnel: [w533 w540] -> w518
              frame True {
                n210 = Multiply(x=w535, y=-1.0) -> (x*y=w532:dbl)
                n211 = call-poly <vilib>:"WPI_RobotDriveHolonomicDrive.vi"("Rotation"=w532, "Y"=0.4 ("X axis value"), "X"=0.0 ("X axis value"), "RobotDriveDevRef"=w536) -> ("RobotDriveDevRef"=w533:T6)  [unwired: 5 in, 2 out]
              }
              frame False {
                n212 = call-poly <vilib>:"WPI_RobotDriveHolonomicDrive.vi"("Rotation"=w539, "Y"=-0.4 ("X axis value"), "X"=0.0 ("X axis value"), "RobotDriveDevRef"=w541) -> ("RobotDriveDevRef"=w540:T6)  [unwired: 5 in, 2 out]
              }
            }
            n213 = call <vilib>:"WPI_EncoderGet.vi"("EncoderDevRef"=w526) -> ("Distance"=w530:dbl, "EncoderDevRef"=w525:T15)  [unwired: 5 in, 4 out]
            n214 = Greater Or Equal?(x=w530, y=1200.0) -> (x >= y?=w528:bool)
          }
        }
        frame #13 {
          w544 = 0.0 ("X")
          n215 = call <vilib>:"WPI_EncoderReset.vi"("EncoderDevRef"=w547) -> ()  [unwired: 9 in, 2 out]
          n216 = call-poly <vilib>:"WPI_RobotDriveHolonomicDrive.vi"("Rotation"=w544, "Y"=w544, "X"=w544, "RobotDriveDevRef"=w546) -> ()  [unwired: 5 in, 3 out]
        }
        frame #14 {
          # "Strafe right"
          n217 = Unbundle By Name(w548) -> ("RobotDriveDevRef"=w550:T6, "EncoderDevRef"=w549:T15)
          n218 = while {
            tunnel: w550 -> [w553]
            tunnel: w549 -> [w552]
            tunnel: [w551] -> _
            stop <- w554 stop-if-true
            n219 = global read "Robot Global Data.vi" "Competition Robot?"() -> (w558:bool)
            n220 = Wait (ms)(milliseconds to wait=u32 30) -> ()  [unwired: 1 out]
            n221 = case shown="False" w558 {
              tunnel: w553 -> [w559 w563]
              frame True {
                n222 = call-poly <vilib>:"WPI_RobotDriveHolonomicDrive.vi"("Rotation"=0.0, "Y"=-1.0 ("X axis value"), "X"=0.0 ("X axis value"), "RobotDriveDevRef"=w559) -> ()  [unwired: 5 in, 3 out]
              }
              frame False {
                n223 = call-poly <vilib>:"WPI_RobotDriveHolonomicDrive.vi"("Rotation"=0.0, "Y"=1.0 ("X axis value"), "X"=0.0 ("X axis value"), "RobotDriveDevRef"=w563) -> ()  [unwired: 5 in, 3 out]
              }
            }
            n224 = call <vilib>:"WPI_EncoderGet.vi"("EncoderDevRef"=w552) -> ("Distance"=w556:dbl, "EncoderDevRef"=w551:T15)  [unwired: 5 in, 4 out]
            n225 = Greater Or Equal?(x=w556, y=-1660.0) -> (x >= y?=w554:bool)
          }
        }
        frame #15 {
          # "Pick up tote #3"
          # "Pick up can"
          n226 = while {
            tunnel: w569 -> [w580]
            tunnel: [w572] -> w567
            tunnel: [w571] -> w568
            stop <- w577 stop-if-true
            n227 = Unbundle By Name(w580) -> ("MotorControlDevRef"=w579:T7, "MotorControlDevRef"=w578:T7, "EncoderDevRef"=w570:T15)
            n228 = while {
              tunnel: w579 -> [w595]
              tunnel: [w594] -> w575
              tunnel: [w593] -> w572
              tunnel: w570 -> [w589]
              stop <- w594 stop-if-true
              n229 = call <vilib>:"WPI_EncoderGet.vi"("EncoderDevRef"=w589) -> ("Distance"=w588:dbl)  [unwired: 5 in, 5 out]
              n230 = call "Auto Front Lift.vi"("Encoder Input"=w588, "Lower Range"=931.0 ("y"), "Upper Range"=951.0 ("y")) -> ("Output"=w590:dbl)  [unwired: 8 in]
              n231 = call <vilib>:"WPI_MotorControlSetOutput.vi"("Output"=w590, "MotorControlDevRef"=w595) -> ("MotorControlDevRef"=w593:T7)  [unwired: 7 in, 2 out]
              n232 = call "Elapsed Time7"() -> ("Time has Elapsed"=w594:bool)  [unwired: 12 in, 7 out]
            }
            n233 = global read "Robot Global Data.vi" "Competition Robot?"() -> (w576:bool)
            n234 = while {
              tunnel: w578 -> [w587]
              tunnel: w576 -> [w585]
              tunnel: [w582] -> w574
              tunnel: [w581] -> w571
              stop <- w582 stop-if-true
              n235 = Select(t=-1.0, s=w585, f=0.0) -> (s? t:f=w586:dbl)
              n236 = call "ARI Time6"() -> ("Time has Elapsed"=w582:bool)  [unwired: 12 in, 7 out]
              n237 = call <vilib>:"WPI_MotorControlSetOutput.vi"("Output"=w586, "MotorControlDevRef"=w587) -> ("MotorControlDevRef"=w581:T7)  [unwired: 7 in, 2 out]
            }
            n238 = And(x=w574, y=w575) -> (x .and. y?=w573:bool)
            n239 = Select(t=w573, s=w576, f=w575) -> (s? t:f=w577:bool)
          }
        }
        frame #16 {
          n240 = call <vilib>:"WPI_MotorControlSetOutput.vi"("Output"=0.0, "MotorControlDevRef"=w598) -> ()  [unwired: 7 in, 3 out]
          n241 = call <vilib>:"WPI_MotorControlSetOutput.vi"("Output"=0.0, "MotorControlDevRef"=w599) -> ()  [unwired: 7 in, 3 out]
        }
        frame #17 {
          n242 = Unbundle By Name(w601) -> ("SimpleGyroDevRef"=w602:T3, "RobotDriveDevRef"=w603:T6)
          n243 = call "WPI_SimpleGyro_Get Angle.vi"("SimpleGyroDevRef"=w602) -> ("Angle"=w604:dbl)  [unwired: 8 in, 2 out]
          n244 = call-poly <vilib>:"WPI_RobotDriveHolonomicDrive.vi"("Rotation"=0.0, "Gyro Angle"=w604, "Y"=0.0, "X"=0.0, "RobotDriveDevRef"=w603) -> ()  [unwired: 4 in, 3 out]
        }
      }
    }
    frame "Both" {
      n245 = call "WPI_SimpleGyro_RefNum Registry Get.vi"("refnum name"="SimpleGyro") -> ("error out"=w637:errorcluster, "SimpleGyroDevRef"=w641:T3)  [unwired: 9 in]
      n246 = call <vilib>:"WPI_RobotDriveRefNum Registry Get.vi"("refnum name"="Four Motors") -> ("error out"=w636:errorcluster, "RobotDriveDevRef"=w640:T6)  [unwired: 1 in, 8 out]
      n247 = call <vilib>:"WPI_EncoderRefNum Registry Get.vi"("refnum name"="Left Front Drive Encoder") -> ("error out"=w635:errorcluster, "EncoderDevRef"=w639:T15)  [unwired: 9 in]
      n248 = call <vilib>:"WPI_MotorControlRefNum Registry Get.vi"("refnum name"="ARI Motor") -> ("error out"=w634:errorcluster, "MotorControlDevRef"=w638:T7)  [unwired: 9 in]
      n249 = call <vilib>:"WPI_RelayRefNum Registry Get.vi"("refnum name"="Clamper Motor") -> ("error out"=w631:errorcluster, "RelayDevRef"=w632:T19)  [unwired: 9 in]
      n250 = call <vilib>:"WPI_MotorControlRefNum Registry Get.vi"("refnum name"="Lifter Motor") -> ("error out"=w628:errorcluster, "MotorControlDevRef"=w629:T7)  [unwired: 9 in]
      n251 = call <vilib>:"WPI_EncoderRefNum Registry Get.vi"("refnum name"="Lifter Motor Encoder") -> ("error out"=w625:errorcluster, "EncoderDevRef"=w626:T15)  [unwired: 9 in]
      n252 = Bundle("SimpleGyroDevRef"=w641, "RobotDriveDevRef"=w640, "EncoderDevRef"=w639, "MotorControlDevRef"=w638, "RelayDevRef"=w632, "MotorControlDevRef"=w629, "EncoderDevRef"=w626) -> (w608:T24)  [unwired: 1 in]
      n253 = Bundle("error out"=w637, "error out"=w636, "error out"=w635, "error out"=w634, "error out"=w631, "error out"=w628, "error out"=w625) -> ()  [unwired: 1 in, 1 out]
      n254 = flat-sequence {
        tunnel: [w652] -> w651
        tunnel: w608 -> [w652]
        tunnel: w651 -> [w657]
        tunnel: [w657] -> w650
        tunnel: [w656] -> w649
        tunnel: w650 -> [w668]
        tunnel: w649 -> [w670]
        tunnel: [w668] -> w623
        tunnel: w623 -> [w672]
        tunnel: [w672] -> w622
        tunnel: [w671] -> w620
        tunnel: w622 -> [w706]
        tunnel: [w706] -> w621
        tunnel: w620 -> [w704]
        tunnel: w621 -> [w708]
        tunnel: [w708] -> w624
        tunnel: [w707] -> w619
        tunnel: w624 -> [w722]
        tunnel: [w722] -> w618
        tunnel: w619 -> [w721]
        tunnel: w618 -> [w724]
        tunnel: [w724] -> w617
        tunnel: [w723] -> w616
        tunnel: w617 -> [w756]
        tunnel: [w756] -> w615
        tunnel: w616 -> [w754]
        tunnel: w615 -> [w758]
        tunnel: [w758] -> w611
        tunnel: [w759] -> w609
        tunnel: w611 -> [w787]
        tunnel: [w787] -> w610
        tunnel: w609 -> [w785]
        tunnel: [w788] -> w648
        tunnel: [w791] -> w647
        tunnel: [w789] -> w646
        tunnel: w610 -> [w788]
        tunnel: w648 -> [w825]
        tunnel: [w825] -> w614
        tunnel: w647 -> [w824]
        tunnel: w646 -> [w823]
        tunnel: w614 -> [w827]
        tunnel: [w827] -> w613
        tunnel: [w826] -> w612
        tunnel: w613 -> [_]
        tunnel: w612 -> [w838]
        frame #0 {
          n255 = Unbundle By Name(w652) -> ("SimpleGyroDevRef"=w654:T3, "EncoderDevRef"=w655:T15, "EncoderDevRef"=w653:T15)
          n256 = call "WPI_SimpleGyro_Reset.vi"("SimpleGyroDevRef"=w654) -> ()  [unwired: 9 in, 2 out]
          n257 = call <vilib>:"WPI_EncoderReset.vi"("EncoderDevRef"=w655) -> ()  [unwired: 9 in, 2 out]
          n258 = call <vilib>:"WPI_EncoderReset.vi"("EncoderDevRef"=w653) -> ()  [unwired: 9 in, 2 out]
        }
        frame #1 {
          # "Picks up Can"
          n259 = while {
            tunnel: w657 -> [w667]
            tunnel: [w665] -> w656
            stop <- w659 stop-if-true
            n260 = Unbundle By Name(w667) -> ("MotorControlDevRef"=w666:T7, "EncoderDevRef"=w658:T15)
            n261 = call <vilib>:"WPI_EncoderGet.vi"("EncoderDevRef"=w658) -> ("Distance"=w663:dbl)  [unwired: 5 in, 5 out]
            n262 = call "Auto Front Lift.vi"("Encoder Input"=w663, "Lower Range"=778.0 ("y"), "Upper Range"=798.0 ("y")) -> ("Output"=w662:dbl)  [unwired: 8 in]
            n263 = Greater?(x=w663, y=800.0) -> (0:w659:bool)
            n264 = call <vilib>:"WPI_MotorControlSetOutput.vi"("Output"=w662, "MotorControlDevRef"=w666) -> ("MotorControlDevRef"=w665:T7)  [unwired: 7 in, 2 out]
          }
        }
        frame #2 {
          n265 = call <vilib>:"WPI_MotorControlSetOutput.vi"("Output"=0.0, "MotorControlDevRef"=w670) -> ()  [unwired: 7 in, 3 out]
        }
        frame #3 {
          # "Drive Forward to pick up tote"
          n266 = Unbundle By Name(w672) -> ("SimpleGyroDevRef"=w673:T3, "RobotDriveDevRef"=w675:T6, "EncoderDevRef"=w674:T15)
          n267 = while {
            tunnel: w675 -> [w685]
            tunnel: w674 -> [w684]
            tunnel: [w683] -> _
            tunnel: w673 -> [w680]
            tunnel: [w676] -> w671
            stop <- w686 stop-if-true
            n268 = global read "Robot Global Data.vi" "Competition Robot?"() -> (w689:bool)
            n269 = call "WPI_SimpleGyro_Get Angle.vi"("SimpleGyroDevRef"=w680) -> ("Angle"=w679:dbl)  [unwired: 8 in, 2 out]
            n270 = call <vilib>:"WPI_EncoderGet.vi"("EncoderDevRef"=w684) -> ("Distance"=w688:dbl, "EncoderDevRef"=w683:T15)  [unwired: 5 in, 4 out]
            n271 = call-poly <vilib>:"PID.vi"("output range"=cluster{"output high":dbl, "output low":dbl} {"output high"=0.2, "output low"=-0.2}, "PID gains"=T2 {"proportional gain (Kc)"=1.0, "integral time (Ti, min)"=0.06, "derivative time (Td, min)"=0.02}, "process variable"=w679, "setpoint"=180.0) -> ("output"=w677:dbl)  [unwired: 6 in, 1 out]
            n272 = case shown="True" w689 {
              tunnel: w685 -> [w694 w701]
              tunnel: w677 -> [w692 w700]
              tunnel: [w691 w698] -> w676
              frame True {
                n273 = Multiply(x=w692, y=-1.0) -> (x*y=w690:dbl)
                n274 = call-poly <vilib>:"WPI_RobotDriveHolonomicDrive.vi"("Rotation"=w690, "Y"=0.28 ("X axis value"), "X"=0.0 ("X axis value"), "RobotDriveDevRef"=w694) -> ("RobotDriveDevRef"=w691:T6)  [unwired: 5 in, 2 out]
              }
              frame False {
                n275 = Multiply(x=w700, y=1.0) -> (x*y=w697:dbl)
                n276 = call-poly <vilib>:"WPI_RobotDriveHolonomicDrive.vi"("Rotation"=w697, "Y"=-0.28 ("X axis value"), "X"=0.0 ("X axis value"), "RobotDriveDevRef"=w701) -> ("RobotDriveDevRef"=w698:T6)  [unwired: 5 in, 2 out]
              }
            }
            n277 = Greater Or Equal?(x=w688, y=420.0) -> (x >= y?=w686:bool)
          }
        }
        frame #4 {
          w705 = 0.0 ("X")
          n278 = call-poly <vilib>:"WPI_RobotDriveHolonomicDrive.vi"("Rotation"=w705, "Y"=w705, "X"=w705, "RobotDriveDevRef"=w704) -> ()  [unwired: 5 in, 3 out]
        }
        frame #5 {
          # "Pick up tote"
          n279 = while {
            tunnel: w708 -> [w718]
            tunnel: [w716] -> w707
            stop <- w710 stop-if-true
            n280 = Unbundle By Name(w718) -> ("MotorControlDevRef"=w717:T7, "EncoderDevRef"=w709:T15)
            n281 = call <vilib>:"WPI_EncoderGet.vi"("EncoderDevRef"=w709) -> ("Distance"=w714:dbl)  [unwired: 5 in, 5 out]
            n282 = call "Auto Front Lift.vi"("Encoder Input"=w714, "Lower Range"=235.0 ("y"), "Upper Range"=255.0 ("y")) -> ("Output"=w713:dbl)  [unwired: 8 in]
            n283 = Greater?(x=w714, y=260.0) -> (0:w710:bool)
            n284 = call <vilib>:"WPI_MotorControlSetOutput.vi"("Output"=w713, "MotorControlDevRef"=w717) -> ("MotorControlDevRef"=w716:T7)  [unwired: 7 in, 2 out]
          }
        }
        frame #6 {
          n285 = Unbundle By Name(w722) -> ("EncoderDevRef"=w719:T15)
          n286 = call <vilib>:"WPI_MotorControlSetOutput.vi"("Output"=0.0, "MotorControlDevRef"=w721) -> ()  [unwired: 7 in, 3 out]
          n287 = call <vilib>:"WPI_EncoderReset.vi"("EncoderDevRef"=w719) -> ()  [unwired: 9 in, 2 out]
        }
        frame #7 {
          # "Strafe Right"
          n288 = Unbundle By Name(w724) -> ("SimpleGyroDevRef"=w725:T3, "RobotDriveDevRef"=w727:T6, "EncoderDevRef"=w726:T15)
          n289 = while {
            tunnel: w727 -> [w737]
            tunnel: w726 -> [w728]
            tunnel: [w736] -> _
            tunnel: w725 -> [w732]
            tunnel: [w729] -> w723
            stop <- w738 stop-if-true
            n290 = global read "Robot Global Data.vi" "Competition Robot?"() -> (w741:bool)
            n291 = call "WPI_SimpleGyro_Get Angle.vi"("SimpleGyroDevRef"=w732) -> ("Angle"=w731:dbl)  [unwired: 8 in, 2 out]
            n292 = call <vilib>:"WPI_EncoderGet.vi"("EncoderDevRef"=w728) -> ("Distance"=w740:dbl, "EncoderDevRef"=w736:T15)  [unwired: 5 in, 4 out]
            n293 = call-poly <vilib>:"PID.vi"("output range"=cluster{"output high":dbl, "output low":dbl} {"output high"=0.2, "output low"=-0.2}, "PID gains"=T2 {"proportional gain (Kc)"=1.2, "integral time (Ti, min)"=0.2, "derivative time (Td, min)"=0.02}, "process variable"=w731, "setpoint"=180.0) -> ("output"=w730:dbl)  [unwired: 6 in, 1 out]
            n294 = case shown="False" w741 {
              tunnel: w737 -> [w746 w751]
              tunnel: w730 -> [w745 w749]
              tunnel: [w743 w750] -> w729
              frame True {
                n295 = Multiply(x=w745, y=-1.0) -> (x*y=w742:dbl)
                n296 = call-poly <vilib>:"WPI_RobotDriveHolonomicDrive.vi"("Rotation"=w742, "Y"=0.0 ("X axis value"), "X"=-0.5 ("X axis value"), "RobotDriveDevRef"=w746) -> ("RobotDriveDevRef"=w743:T6)  [unwired: 5 in, 2 out]
              }
              frame False {
                n297 = call-poly <vilib>:"WPI_RobotDriveHolonomicDrive.vi"("Rotation"=w749, "Y"=0.0 ("X axis value"), "X"=0.5 ("X axis value"), "RobotDriveDevRef"=w751) -> ("RobotDriveDevRef"=w750:T6)  [unwired: 5 in, 2 out]
              }
            }
            n298 = Greater Or Equal?(x=w740, y=100.0) -> (x >= y?=w738:bool)
          }
        }
        frame #8 {
          w755 = 0.0 ("X")
          n299 = Unbundle By Name(w756) -> ("EncoderDevRef"=w757:T15)
          n300 = call-poly <vilib>:"WPI_RobotDriveHolonomicDrive.vi"("Rotation"=w755, "Y"=w755, "X"=w755, "RobotDriveDevRef"=w754) -> ()  [unwired: 5 in, 3 out]
          n301 = call <vilib>:"WPI_EncoderReset.vi"("EncoderDevRef"=w757) -> ()  [unwired: 9 in, 2 out]
        }
        frame #9 {
          # "Turn 90 degrees"
          n302 = Unbundle By Name(w758) -> ("SimpleGyroDevRef"=w761:T3, "RobotDriveDevRef"=w760:T6)
          n303 = while {
            tunnel: w761 -> [w769]
            tunnel: w760 -> [w768]
            tunnel: [w762] -> w759
            stop <- w770 stop-if-true
            n304 = global read "Robot Global Data.vi" "Competition Robot?"() -> (w771:bool)
            n305 = call "WPI_SimpleGyro_Get Angle.vi"("SimpleGyroDevRef"=w769) -> ("Angle"=w763:dbl)  [unwired: 8 in, 2 out]
            n306 = call-poly <vilib>:"PID.vi"("output range"=cluster{"output high":dbl, "output low":dbl} {"output high"=0.45, "output low"=-0.45}, "PID gains"=T2 {"proportional gain (Kc)"=1.0, "integral time (Ti, min)"=0.001, "derivative time (Td, min)"=0.0}, "process variable"=w763, "setpoint"=90.0) -> ("output"=w764:dbl)  [unwired: 6 in, 1 out]
            n307 = case shown="False" w771 {
              tunnel: w768 -> [w777 w782]
              tunnel: w764 -> [w776 w781]
              tunnel: [w773 w780] -> w762
              frame True {
                n308 = Multiply(x=w776, y=-1.0) -> (x*y=w774:dbl)
                n309 = call-poly <vilib>:"WPI_RobotDriveHolonomicDrive.vi"("Rotation"=w774, "Y"=0.0 ("X axis value"), "X"=0.0 ("X axis value"), "RobotDriveDevRef"=w777) -> ("RobotDriveDevRef"=w773:T6)  [unwired: 5 in, 2 out]
              }
              frame False {
                n310 = call-poly <vilib>:"WPI_RobotDriveHolonomicDrive.vi"("Rotation"=w781, "Y"=0.0 ("X axis value"), "X"=0.0 ("X axis value"), "RobotDriveDevRef"=w782) -> ("RobotDriveDevRef"=w780:T6)  [unwired: 5 in, 2 out]
              }
            }
            n311 = Greater Or Equal?(x=w763, y=85.0) -> (x >= y?=w770:bool)
          }
        }
        frame #10 {
          w786 = 0.0 ("X")
          n312 = call-poly <vilib>:"WPI_RobotDriveHolonomicDrive.vi"("Rotation"=w786, "Y"=w786, "X"=w786, "RobotDriveDevRef"=w785) -> ()  [unwired: 5 in, 3 out]
        }
        frame #11 {
          # "Drive forward"
          n313 = Unbundle By Name(w788) -> ("SimpleGyroDevRef"=w790:T3, "RobotDriveDevRef"=w793:T6, "EncoderDevRef"=w792:T15)
          n314 = while {
            tunnel: w793 -> [w803]
            tunnel: w792 -> [w802]
            tunnel: [w801] -> w791
            tunnel: w790 -> [w798]
            tunnel: [w794] -> w789
            stop <- w804 stop-if-true
            n315 = global read "Robot Global Data.vi" "Competition Robot?"() -> (w807:bool)
            n316 = call "WPI_SimpleGyro_Get Angle.vi"("SimpleGyroDevRef"=w798) -> ("Angle"=w797:dbl)  [unwired: 8 in, 2 out]
            n317 = call <vilib>:"WPI_EncoderGet.vi"("EncoderDevRef"=w802) -> ("Distance"=w806:dbl, "EncoderDevRef"=w801:T15)  [unwired: 5 in, 4 out]
            n318 = call-poly <vilib>:"PID.vi"("output range"=cluster{"output high":dbl, "output low":dbl} {"output high"=0.2, "output low"=-0.2}, "PID gains"=T2 {"proportional gain (Kc)"=1.0, "integral time (Ti, min)"=0.06, "derivative time (Td, min)"=0.02}, "process variable"=w797, "setpoint"=180.0) -> ("output"=w795:dbl)  [unwired: 6 in, 1 out]
            n319 = case shown="True" w807 {
              tunnel: w803 -> [w812 w819]
              tunnel: w795 -> [w810 w818]
              tunnel: [w809 w816] -> w794
              frame True {
                n320 = Multiply(x=w810, y=-1.0) -> (x*y=w808:dbl)
                n321 = call-poly <vilib>:"WPI_RobotDriveHolonomicDrive.vi"("Rotation"=w808, "Y"=0.28 ("X axis value"), "X"=0.0 ("X axis value"), "RobotDriveDevRef"=w812) -> ("RobotDriveDevRef"=w809:T6)  [unwired: 5 in, 2 out]
              }
              frame False {
                n322 = Multiply(x=w818, y=1.0) -> (x*y=w815:dbl)
                n323 = call-poly <vilib>:"WPI_RobotDriveHolonomicDrive.vi"("Rotation"=w815, "Y"=-0.28 ("X axis value"), "X"=0.0 ("X axis value"), "RobotDriveDevRef"=w819) -> ("RobotDriveDevRef"=w816:T6)  [unwired: 5 in, 2 out]
              }
            }
            n324 = Greater Or Equal?(x=w806, y=1460.0) -> (x >= y?=w804:bool)
          }
        }
        frame #12 {
          w822 = 0.0 ("X")
          n325 = call <vilib>:"WPI_EncoderReset.vi"("EncoderDevRef"=w824) -> ()  [unwired: 9 in, 2 out]
          n326 = call-poly <vilib>:"WPI_RobotDriveHolonomicDrive.vi"("Rotation"=w822, "Y"=w822, "X"=w822, "RobotDriveDevRef"=w823) -> ()  [unwired: 5 in, 3 out]
        }
        frame #13 {
          # "Drops"
          n327 = while {
            tunnel: w827 -> [w837]
            tunnel: [w835] -> w826
            stop <- w829 stop-if-true
            n328 = Unbundle By Name(w837) -> ("MotorControlDevRef"=w836:T7, "EncoderDevRef"=w828:T15)
            n329 = call <vilib>:"WPI_EncoderGet.vi"("EncoderDevRef"=w828) -> ("Distance"=w833:dbl)  [unwired: 5 in, 5 out]
            n330 = call "Auto Front Lift.vi"("Encoder Input"=w833, "Lower Range"=-798.0 ("y"), "Upper Range"=-778.0 ("y")) -> ("Output"=w832:dbl)  [unwired: 8 in]
            n331 = Less Or Equal?(x=w833, y=-800.0) -> (x <= y?=w829:bool)
            n332 = call <vilib>:"WPI_MotorControlSetOutput.vi"("Output"=w832, "MotorControlDevRef"=w836) -> ("MotorControlDevRef"=w835:T7)  [unwired: 7 in, 2 out]
          }
        }
        frame #14 {
          n333 = call <vilib>:"WPI_MotorControlSetOutput.vi"("Output"=0.0, "MotorControlDevRef"=w838) -> ()  [unwired: 7 in, 3 out]
        }
      }
    }
    frame "Tote and Can" {
      n334 = call "WPI_SimpleGyro_RefNum Registry Get.vi"("refnum name"="SimpleGyro") -> ("error out"=w886:errorcluster, "SimpleGyroDevRef"=w890:T3)  [unwired: 9 in]
      n335 = call <vilib>:"WPI_RobotDriveRefNum Registry Get.vi"("refnum name"="Four Motors") -> ("error out"=w885:errorcluster, "RobotDriveDevRef"=w889:T6)  [unwired: 1 in, 8 out]
      n336 = call <vilib>:"WPI_EncoderRefNum Registry Get.vi"("refnum name"="Left Front Drive Encoder") -> ("error out"=w884:errorcluster, "EncoderDevRef"=w888:T15)  [unwired: 9 in]
      n337 = call <vilib>:"WPI_MotorControlRefNum Registry Get.vi"("refnum name"="ARI Motor") -> ("error out"=w883:errorcluster, "MotorControlDevRef"=w887:T7)  [unwired: 9 in]
      n338 = call <vilib>:"WPI_RelayRefNum Registry Get.vi"("refnum name"="Clamper Motor") -> ("error out"=w880:errorcluster, "RelayDevRef"=w881:T19)  [unwired: 9 in]
      n339 = call <vilib>:"WPI_MotorControlRefNum Registry Get.vi"("refnum name"="Lifter Motor") -> ("error out"=w877:errorcluster, "MotorControlDevRef"=w878:T7)  [unwired: 9 in]
      n340 = call <vilib>:"WPI_EncoderRefNum Registry Get.vi"("refnum name"="Lifter Motor Encoder") -> ("error out"=w874:errorcluster, "EncoderDevRef"=w875:T15)  [unwired: 9 in]
      n341 = Bundle("SimpleGyroDevRef"=w890, "RobotDriveDevRef"=w889, "EncoderDevRef"=w888, "MotorControlDevRef"=w887, "RelayDevRef"=w881, "MotorControlDevRef"=w878, "EncoderDevRef"=w875) -> (w873:T24)  [unwired: 1 in]
      n342 = Bundle("error out"=w886, "error out"=w885, "error out"=w884, "error out"=w883, "error out"=w880, "error out"=w877, "error out"=w874) -> ()  [unwired: 1 in, 1 out]
      n343 = flat-sequence {
        tunnel: w873 -> [w897]
        tunnel: [w897] -> w871
        tunnel: w871 -> [w901]
        tunnel: [w901] -> w861
        tunnel: [w903] -> w872
        tunnel: [w904] -> w867
        tunnel: w861 -> [w903]
        tunnel: w872 -> [w913]
        tunnel: [w913] -> w870
        tunnel: w867 -> [w912]
        tunnel: w870 -> [w916]
        tunnel: [w916] -> w869
        tunnel: [w915] -> w868
        tunnel: w869 -> [w943]
        tunnel: w868 -> [w944]
        tunnel: [w943] -> w847
        tunnel: w847 -> [w948]
        tunnel: [w948] -> w846
        tunnel: [w947] -> w844
        tunnel: [w946] -> w843
        tunnel: w846 -> [w980]
        tunnel: [w980] -> w845
        tunnel: w844 -> [w978]
        tunnel: w843 -> [w977]
        tunnel: w845 -> [w983]
        tunnel: [w983] -> w860
        tunnel: [w982] -> w859
        tunnel: [w981] -> w858
        tunnel: w860 -> [w1012]
        tunnel: w859 -> [w1014]
        tunnel: w858 -> [w1013]
        tunnel: [w1012] -> w842
        tunnel: [w1016] -> w854
        tunnel: w842 -> [w1016]
        tunnel: w854 -> [w1021]
        tunnel: [w1021] -> w857
        tunnel: [w1019] -> w856
        tunnel: [w1018] -> w855
        tunnel: w857 -> [w1049]
        tunnel: [w1049] -> w866
        tunnel: w856 -> [w1051]
        tunnel: w855 -> [w1050]
        tunnel: w866 -> [w1055]
        tunnel: [w1055] -> w896
        tunnel: [w1054] -> w895
        tunnel: [w1053] -> w853
        tunnel: w896 -> [w1069]
        tunnel: [w1069] -> w865
        tunnel: w895 -> [w1071]
        tunnel: w853 -> [w1068]
        tunnel: w865 -> [w1075]
        tunnel: [w1075] -> w864
        tunnel: [w1072] -> w852
        tunnel: w864 -> [w1101]
        tunnel: [w1101] -> w851
        tunnel: w852 -> [w1099]
        tunnel: w851 -> [w1103]
        tunnel: [w1103] -> w850
        tunnel: [w1102] -> w848
        tunnel: w850 -> [w1133]
        tunnel: [w1133] -> w849
        tunnel: w848 -> [w1131]
        tunnel: w849 -> [w1135]
        tunnel: [w1135] -> w863
        tunnel: [w1136] -> w862
        tunnel: [w1134] -> w841
        tunnel: w863 -> [w1150]
        tunnel: w862 -> [w1152]
        tunnel: w841 -> [w1149]
        tunnel: [w1150] -> w840
        tunnel: [w1153] -> _
        tunnel: w840 -> [w1153]
        frame #0 {
          n344 = Unbundle By Name(w897) -> ("SimpleGyroDevRef"=w899:T3, "EncoderDevRef"=w900:T15, "EncoderDevRef"=w898:T15)
          n345 = call "WPI_SimpleGyro_Reset.vi"("SimpleGyroDevRef"=w899) -> ()  [unwired: 9 in, 2 out]
          n346 = call <vilib>:"WPI_EncoderReset.vi"("EncoderDevRef"=w900) -> ()  [unwired: 9 in, 2 out]
          n347 = call <vilib>:"WPI_EncoderReset.vi"("EncoderDevRef"=w898) -> ()  [unwired: 9 in, 2 out]
        }
        frame #1 {
          # "Delay"
          n348 = while {
            stop <- w902 stop-if-true
            n349 = call "Clamper Time2"() -> ("Time has Elapsed"=w902:bool)  [unwired: 12 in, 7 out]
          }
        }
        frame #2 {
          # "Picks up Can"
          n350 = while {
            tunnel: w903 -> [w908]
            tunnel: [w906] -> w904
            stop <- w905 stop-if-true
            n351 = Unbundle By Name(w908) -> ("MotorControlDevRef"=w907:T7)
            n352 = call "Clamper Time5"() -> ("Time has Elapsed"=w905:bool)  [unwired: 12 in, 7 out]
            n353 = call "Auto Front Lift.vi"("Lower Range"=778.0 ("y"), "Upper Range"=798.0 ("y")) -> ("Output"=w911:dbl)  [unwired: 9 in]
            n354 = call <vilib>:"WPI_MotorControlSetOutput.vi"("Output"=w911, "MotorControlDevRef"=w907) -> ("MotorControlDevRef"=w906:T7)  [unwired: 7 in, 2 out]
          }
        }
        frame #3 {
          n355 = call <vilib>:"WPI_MotorControlSetOutput.vi"("Output"=0.0, "MotorControlDevRef"=w912) -> ()  [unwired: 7 in, 3 out]
        }
        frame #4 {
          # "Clockwise 90 Degrees"
          n356 = Unbundle By Name(w916) -> ("SimpleGyroDevRef"=w918:T3, "RobotDriveDevRef"=w917:T6)
          n357 = while {
            tunnel: w918 -> [w926]
            tunnel: w917 -> [w925]
            tunnel: [w919] -> w915
            stop <- w927 stop-if-true
            n358 = global read "Robot Global Data.vi" "Competition Robot?"() -> (w928:bool)
            n359 = call "WPI_SimpleGyro_Get Angle.vi"("SimpleGyroDevRef"=w926) -> ("Angle"=w920:dbl)  [unwired: 8 in, 2 out]
            n360 = call-poly <vilib>:"PID.vi"("output range"=cluster{"output high":dbl, "output low":dbl} {"output high"=0.4, "output low"=-0.4}, "PID gains"=T2 {"proportional gain (Kc)"=1.0, "integral time (Ti, min)"=0.002, "derivative time (Td, min)"=0.0}, "process variable"=w920, "setpoint"=90.0) -> ("output"=w921:dbl)  [unwired: 6 in, 1 out]
            n361 = case shown="False" w928 {
              tunnel: w925 -> [w934 w939]
              tunnel: w921 -> [w933 w938]
              tunnel: [w930 w937] -> w919
              frame True {
                n362 = Multiply(x=w933, y=-1.0) -> (x*y=w931:dbl)
                n363 = call-poly <vilib>:"WPI_RobotDriveHolonomicDrive.vi"("Rotation"=w931, "Y"=0.0 ("X axis value"), "X"=0.0 ("X axis value"), "RobotDriveDevRef"=w934) -> ("RobotDriveDevRef"=w930:T6)  [unwired: 5 in, 2 out]
              }
              frame False {
                n364 = call-poly <vilib>:"WPI_RobotDriveHolonomicDrive.vi"("Rotation"=w938, "Y"=0.0 ("X axis value"), "X"=0.0 ("X axis value"), "RobotDriveDevRef"=w939) -> ("RobotDriveDevRef"=w937:T6)  [unwired: 5 in, 2 out]
              }
            }
            n365 = Greater Or Equal?(x=w920, y=86.0) -> (x >= y?=w927:bool)
          }
        }
        frame #5 {
          w945 = 0.0 ("X")
          n366 = Unbundle By Name(w943) -> ("EncoderDevRef"=w942:T15)
          n367 = call-poly <vilib>:"WPI_RobotDriveHolonomicDrive.vi"("Rotation"=w945, "Y"=w945, "X"=w945, "RobotDriveDevRef"=w944) -> ()  [unwired: 5 in, 3 out]
          n368 = call <vilib>:"WPI_EncoderReset.vi"("EncoderDevRef"=w942) -> ()  [unwired: 9 in, 2 out]
        }
        frame #6 {
          # "Drive backward"
          n369 = Unbundle By Name(w948) -> ("SimpleGyroDevRef"=w949:T3, "RobotDriveDevRef"=w951:T6, "EncoderDevRef"=w950:T15)
          n370 = while {
            tunnel: w951 -> [w963]
            tunnel: w950 -> [w954]
            tunnel: [w962] -> w947
            tunnel: w949 -> [w958]
            tunnel: [w955] -> w946
            stop <- w964 stop-if-true
            n371 = global read "Robot Global Data.vi" "Competition Robot?"() -> (w966:bool)
            n372 = call "WPI_SimpleGyro_Get Angle.vi"("SimpleGyroDevRef"=w958) -> ("Angle"=w957:dbl)  [unwired: 8 in, 2 out]
            n373 = call <vilib>:"WPI_EncoderGet.vi"("EncoderDevRef"=w954) -> ("Distance"=w952:dbl, "EncoderDevRef"=w962:T15)  [unwired: 5 in, 4 out]
            n374 = call-poly <vilib>:"SD Write Value.vi"("Numeric"=w952, "Name"="Wheel Encoder") -> ()  [unwired: 8 in, 2 out]
            n375 = call-poly <vilib>:"PID.vi"("output range"=cluster{"output high":dbl, "output low":dbl} {"output high"=0.2, "output low"=-0.2}, "PID gains"=T2 {"proportional gain (Kc)"=1.2, "integral time (Ti, min)"=0.2, "derivative time (Td, min)"=0.02}, "process variable"=w957, "setpoint"=180.0) -> ("output"=w956:dbl)  [unwired: 6 in, 1 out]
            n376 = case shown="False" w966 {
              tunnel: w963 -> [w970 w975]
              tunnel: w956 -> [w967 w973]
              tunnel: [w969 w974] -> w955
              frame True {
                n377 = call-poly <vilib>:"WPI_RobotDriveHolonomicDrive.vi"("Rotation"=0.0 ("X axis value"), "Y"=w967, "X"=0.5 ("X axis value"), "RobotDriveDevRef"=w970) -> ("RobotDriveDevRef"=w969:T6)  [unwired: 5 in, 2 out]
              }
              frame False {
                n378 = call-poly <vilib>:"WPI_RobotDriveHolonomicDrive.vi"("Rotation"=0.0, "Y"=w973, "X"=-0.5 ("X axis value"), "RobotDriveDevRef"=w975) -> ("RobotDriveDevRef"=w974:T6)  [unwired: 5 in, 2 out]
              }
            }
            n379 = Less Or Equal?(x=w952, y=-300.0) -> (x <= y?=w964:bool)
          }
        }
        frame #7 {
          w979 = 0.0 ("X")
          n380 = call <vilib>:"WPI_EncoderReset.vi"("EncoderDevRef"=w978) -> ()  [unwired: 9 in, 2 out]
          n381 = call-poly <vilib>:"WPI_RobotDriveHolonomicDrive.vi"("Rotation"=w979, "Y"=w979, "X"=w979, "RobotDriveDevRef"=w977) -> ()  [unwired: 5 in, 3 out]
        }
        frame #8 {
          # "Strafe Left"
          n382 = Unbundle By Name(w983) -> ("SimpleGyroDevRef"=w984:T3, "RobotDriveDevRef"=w986:T6, "EncoderDevRef"=w985:T15)
          n383 = while {
            tunnel: w986 -> [w998]
            tunnel: w985 -> [w989]
            tunnel: [w997] -> w981
            tunnel: w984 -> [w993]
            tunnel: [w990] -> w982
            stop <- w999 stop-if-true
            n384 = global read "Robot Global Data.vi" "Competition Robot?"() -> (w1001:bool)
            n385 = call "WPI_SimpleGyro_Get Angle.vi"("SimpleGyroDevRef"=w993) -> ("Angle"=w992:dbl)  [unwired: 8 in, 2 out]
            n386 = call <vilib>:"WPI_EncoderGet.vi"("EncoderDevRef"=w989) -> ("Distance"=w987:dbl, "EncoderDevRef"=w997:T15)  [unwired: 5 in, 4 out]
            n387 = call-poly <vilib>:"SD Write Value.vi"("Numeric"=w987, "Name"="Wheel Encoder") -> ()  [unwired: 8 in, 2 out]
            n388 = call-poly <vilib>:"PID.vi"("output range"=cluster{"output high":dbl, "output low":dbl} {"output high"=0.2, "output low"=-0.2}, "PID gains"=T2 {"proportional gain (Kc)"=1.2, "integral time (Ti, min)"=0.2, "derivative time (Td, min)"=0.02}, "process variable"=w992, "setpoint"=180.0) -> ("output"=w991:dbl)  [unwired: 6 in, 1 out]
            n389 = case shown="True" w1001 {
              tunnel: w998 -> [w1004 w1009]
              tunnel: w991 -> [w1002 w1007]
              tunnel: [w1003 w1008] -> w990
              frame True {
                n390 = call-poly <vilib>:"WPI_RobotDriveHolonomicDrive.vi"("Rotation"=w1002, "Y"=0.0 ("X axis value"), "X"=0.5 ("X axis value"), "RobotDriveDevRef"=w1004) -> ("RobotDriveDevRef"=w1003:T6)  [unwired: 5 in, 2 out]
              }
              frame False {
                n391 = call-poly <vilib>:"WPI_RobotDriveHolonomicDrive.vi"("Rotation"=w1007, "Y"=0.0 ("X axis value"), "X"=-0.5 ("X axis value"), "RobotDriveDevRef"=w1009) -> ("RobotDriveDevRef"=w1008:T6)  [unwired: 5 in, 2 out]
              }
            }
            n392 = Less Or Equal?(x=w987, y=-475.0) -> (x <= y?=w999:bool)
          }
        }
        frame #9 {
          w1015 = 0.0 ("X")
          n393 = call <vilib>:"WPI_EncoderReset.vi"("EncoderDevRef"=w1013) -> ()  [unwired: 9 in, 2 out]
          n394 = call-poly <vilib>:"WPI_RobotDriveHolonomicDrive.vi"("Rotation"=w1015, "Y"=w1015, "X"=w1015, "RobotDriveDevRef"=w1014) -> ()  [unwired: 5 in, 3 out]
        }
        frame #10 {
          n395 = while {
            stop <- w1017 stop-if-true
            n396 = call "Clamper Time4"() -> ("Time has Elapsed"=w1017:bool)  [unwired: 12 in, 7 out]
          }
        }
        frame #11 {
          # "Love-tap the tote"
          n397 = Unbundle By Name(w1021) -> ("SimpleGyroDevRef"=w1022:T3, "RobotDriveDevRef"=w1020:T6, "EncoderDevRef"=w1023:T15)
          n398 = while {
            tunnel: w1020 -> [w1035]
            tunnel: w1023 -> [w1026]
            tunnel: [w1034] -> w1018
            tunnel: w1022 -> [w1030]
            tunnel: [w1027] -> w1019
            stop <- w1036 stop-if-true
            n399 = global read "Robot Global Data.vi" "Competition Robot?"() -> (w1038:bool)
            n400 = call "WPI_SimpleGyro_Get Angle.vi"("SimpleGyroDevRef"=w1030) -> ("Angle"=w1029:dbl)  [unwired: 8 in, 2 out]
            n401 = call <vilib>:"WPI_EncoderGet.vi"("EncoderDevRef"=w1026) -> ("Distance"=w1024:dbl, "EncoderDevRef"=w1034:T15)  [unwired: 5 in, 4 out]
            n402 = call-poly <vilib>:"SD Write Value.vi"("Numeric"=w1024, "Name"="Wheel Encoder") -> ()  [unwired: 8 in, 2 out]
            n403 = call-poly <vilib>:"PID.vi"("output range"=cluster{"output high":dbl, "output low":dbl} {"output high"=0.2, "output low"=-0.2}, "PID gains"=T2 {"proportional gain (Kc)"=1.2, "integral time (Ti, min)"=0.06, "derivative time (Td, min)"=0.0}, "process variable"=w1029, "setpoint"=88.0) -> ("output"=w1028:dbl)  [unwired: 6 in, 1 out]
            n404 = case shown="False" w1038 {
              tunnel: w1035 -> [w1041 w1046]
              tunnel: w1028 -> [w1039 w1044]
              tunnel: [w1040 w1045] -> w1027
              frame True {
                n405 = call-poly <vilib>:"WPI_RobotDriveHolonomicDrive.vi"("Rotation"=w1039, "Y"=-0.2 ("X axis value"), "X"=0.0 ("X axis value"), "RobotDriveDevRef"=w1041) -> ("RobotDriveDevRef"=w1040:T6)  [unwired: 5 in, 2 out]
              }
              frame False {
                n406 = call-poly <vilib>:"WPI_RobotDriveHolonomicDrive.vi"("Rotation"=w1044, "Y"=-0.15 ("X axis value"), "X"=0.0 ("X axis value"), "RobotDriveDevRef"=w1046) -> ("RobotDriveDevRef"=w1045:T6)  [unwired: 5 in, 2 out]
              }
            }
            n407 = Greater Or Equal?(x=w1024, y=250.0) -> (x >= y?=w1036:bool)
          }
        }
        frame #12 {
          w1052 = 0.0 ("X")
          n408 = call <vilib>:"WPI_EncoderReset.vi"("EncoderDevRef"=w1050) -> ()  [unwired: 9 in, 2 out]
          n409 = call-poly <vilib>:"WPI_RobotDriveHolonomicDrive.vi"("Rotation"=w1052, "Y"=w1052, "X"=w1052, "RobotDriveDevRef"=w1051) -> ()  [unwired: 5 in, 3 out]
        }
        frame #13 {
          # "Pick up tote"
          n410 = while {
            tunnel: w1055 -> [w1067]
            tunnel: [w1065] -> w1054
            tunnel: [w1056] -> w1053
            stop <- w1063 stop-if-true
            n411 = Unbundle By Name(w1067) -> ("MotorControlDevRef"=w1066:T7, "EncoderDevRef"=w1062:T15)
            n412 = call <vilib>:"WPI_EncoderGet.vi"("EncoderDevRef"=w1062) -> ("Distance"=w1061:dbl, "EncoderDevRef"=w1056:T15)  [unwired: 5 in, 4 out]
            n413 = call-poly <vilib>:"PID.vi"("output range"=cluster{"output high":dbl, "output low":dbl} {"output high"=1.0, "output low"=-1.0}, "PID gains"=T2 {"proportional gain (Kc)"=1.0, "integral time (Ti, min)"=0.001, "derivative time (Td, min)"=0.0}, "process variable"=w1061, "setpoint"=500.0) -> ("output"=w1060:dbl)  [unwired: 6 in, 1 out]
            n414 = Greater?(x=w1061, y=495.0) -> (0:w1063:bool)
            n415 = call <vilib>:"WPI_MotorControlSetOutput.vi"("Output"=w1060, "MotorControlDevRef"=w1066) -> ("MotorControlDevRef"=w1065:T7)  [unwired: 7 in, 2 out]
          }
        }
        frame #14 {
          n416 = call <vilib>:"WPI_EncoderReset.vi"("EncoderDevRef"=w1068) -> ()  [unwired: 9 in, 2 out]
          n417 = call <vilib>:"WPI_MotorControlSetOutput.vi"("Output"=0.0, "MotorControlDevRef"=w1071) -> ()  [unwired: 7 in, 3 out]
        }
        frame #15 {
          # "Rotate Clockwise 90 Degrees"
          n418 = Unbundle By Name(w1075) -> ("SimpleGyroDevRef"=w1074:T3, "RobotDriveDevRef"=w1073:T6)  [unwired: 1 out]
          n419 = while {
            tunnel: [w1078] -> w1072
            tunnel: w1074 -> [w1077]
            tunnel: w1073 -> [w1076]
            stop <- w1084 stop-if-true
            n420 = global read "Robot Global Data.vi" "Competition Robot?"() -> (w1085:bool)
            n421 = call "WPI_SimpleGyro_Get Angle.vi"("SimpleGyroDevRef"=w1077) -> ("Angle"=w1079:dbl)  [unwired: 8 in, 2 out]
            n422 = call-poly <vilib>:"PID.vi"("output range"=cluster{"output high":dbl, "output low":dbl} {"output high"=0.4, "output low"=-0.4}, "PID gains"=T2 {"proportional gain (Kc)"=1.0, "integral time (Ti, min)"=0.002, "derivative time (Td, min)"=0.0}, "process variable"=w1079, "setpoint"=180.0) -> ("output"=w1080:dbl)  [unwired: 6 in, 1 out]
            n423 = case shown="True" w1085 {
              tunnel: w1080 -> [w1087 w1096]
              tunnel: [w1089 w1095] -> w1078
              tunnel: w1076 -> [w1088 w1094]
              frame True {
                n424 = Multiply(x=w1087, y=-1.0) -> (x*y=w1090:dbl)
                n425 = call-poly <vilib>:"WPI_RobotDriveHolonomicDrive.vi"("Rotation"=w1090, "Y"=0.0 ("X axis value"), "X"=0.0 ("X axis value"), "RobotDriveDevRef"=w1088) -> ("RobotDriveDevRef"=w1089:T6)  [unwired: 5 in, 2 out]
              }
              frame False {
                n426 = call-poly <vilib>:"WPI_RobotDriveHolonomicDrive.vi"("Rotation"=w1096, "Y"=0.0 ("X axis value"), "X"=0.0 ("X axis value"), "RobotDriveDevRef"=w1094) -> ("RobotDriveDevRef"=w1095:T6)  [unwired: 5 in, 2 out]
              }
            }
            n427 = Greater Or Equal?(x=w1079, y=178.0) -> (x >= y?=w1084:bool)
          }
        }
        frame #16 {
          w1100 = 0.0 ("X")
          n428 = call-poly <vilib>:"WPI_RobotDriveHolonomicDrive.vi"("Rotation"=w1100, "Y"=w1100, "X"=w1100, "RobotDriveDevRef"=w1099) -> ()  [unwired: 5 in, 3 out]
        }
        frame #17 {
          # "Drive forward"
          n429 = Unbundle By Name(w1103) -> ("SimpleGyroDevRef"=w1105:T3, "RobotDriveDevRef"=w1104:T6, "EncoderDevRef"=w1106:T15)
          n430 = while {
            tunnel: w1104 -> [w1117]
            tunnel: w1106 -> [w1108]
            tunnel: [w1116] -> _
            tunnel: w1105 -> [w1112]
            tunnel: [w1109] -> w1102
            stop <- w1118 stop-if-true
            n431 = global read "Robot Global Data.vi" "Competition Robot?"() -> (w1120:bool)
            n432 = call "WPI_SimpleGyro_Get Angle.vi"("SimpleGyroDevRef"=w1112) -> ("Angle"=w1111:dbl)  [unwired: 8 in, 2 out]
            n433 = call <vilib>:"WPI_EncoderGet.vi"("EncoderDevRef"=w1108) -> ("Distance"=w1107:dbl, "EncoderDevRef"=w1116:T15)  [unwired: 5 in, 4 out]
            n434 = call-poly <vilib>:"PID.vi"("output range"=cluster{"output high":dbl, "output low":dbl} {"output high"=0.3, "output low"=-0.3}, "PID gains"=T2 {"proportional gain (Kc)"=1.2, "integral time (Ti, min)"=0.01, "derivative time (Td, min)"=0.0}, "process variable"=w1111, "setpoint"=180.0) -> ("output"=w1110:dbl)  [unwired: 6 in, 1 out]
            n435 = case shown="False" w1120 {
              tunnel: w1117 -> [w1123 w1128]
              tunnel: w1110 -> [w1121 w1126]
              tunnel: [w1122 w1127] -> w1109
              frame True {
                n436 = call-poly <vilib>:"WPI_RobotDriveHolonomicDrive.vi"("Rotation"=w1121, "Y"=-0.2 ("X axis value"), "X"=0.0 ("X axis value"), "RobotDriveDevRef"=w1123) -> ("RobotDriveDevRef"=w1122:T6)  [unwired: 5 in, 2 out]
              }
              frame False {
                n437 = call-poly <vilib>:"WPI_RobotDriveHolonomicDrive.vi"("Rotation"=w1126, "Y"=-0.5 ("X axis value"), "X"=0.0 ("X axis value"), "RobotDriveDevRef"=w1128) -> ("RobotDriveDevRef"=w1127:T6)  [unwired: 5 in, 2 out]
              }
            }
            n438 = Greater Or Equal?(x=w1107, y=380.0) -> (x >= y?=w1118:bool)
          }
        }
        frame #18 {
          w1132 = 0.0 ("X")
          n439 = call-poly <vilib>:"WPI_RobotDriveHolonomicDrive.vi"("Rotation"=w1132, "Y"=w1132, "X"=w1132, "RobotDriveDevRef"=w1131) -> ()  [unwired: 5 in, 3 out]
        }
        frame #19 {
          # "Drops"
          n440 = while {
            tunnel: w1135 -> [w1148]
            tunnel: [w1146] -> w1136
            tunnel: [w1137] -> w1134
            stop <- w1144 stop-if-true
            n441 = Unbundle By Name(w1148) -> ("MotorControlDevRef"=w1147:T7, "EncoderDevRef"=w1143:T15)
            n442 = call <vilib>:"WPI_EncoderGet.vi"("EncoderDevRef"=w1143) -> ("Distance"=w1142:dbl, "EncoderDevRef"=w1137:T15)  [unwired: 5 in, 4 out]
            n443 = call-poly <vilib>:"PID.vi"("output range"=cluster{"output high":dbl, "output low":dbl} {"output high"=1.0, "output low"=-1.0}, "PID gains"=T2 {"proportional gain (Kc)"=1.0, "integral time (Ti, min)"=0.001, "derivative time (Td, min)"=0.0}, "process variable"=w1142, "setpoint"=-500.0) -> ("output"=w1141:dbl)  [unwired: 6 in, 1 out]
            n444 = Less?(x=w1142, y=-215.0) -> (x < y?=w1144:bool)
            n445 = call <vilib>:"WPI_MotorControlSetOutput.vi"("Output"=w1141, "MotorControlDevRef"=w1147) -> ("MotorControlDevRef"=w1146:T7)  [unwired: 7 in, 2 out]
          }
        }
        frame #20 {
          n446 = call <vilib>:"WPI_EncoderReset.vi"("EncoderDevRef"=w1149) -> ()  [unwired: 9 in, 2 out]
          n447 = call <vilib>:"WPI_MotorControlSetOutput.vi"("Output"=0.0, "MotorControlDevRef"=w1152) -> ()  [unwired: 7 in, 3 out]
        }
        frame #21 {
          n448 = Unbundle By Name(w1153) -> ("SimpleGyroDevRef"=w1154:T3, "RobotDriveDevRef"=w1155:T6)
          n449 = call "WPI_SimpleGyro_Get Angle.vi"("SimpleGyroDevRef"=w1154) -> ("Angle"=w1156:dbl)  [unwired: 8 in, 2 out]
          n450 = call-poly <vilib>:"WPI_RobotDriveHolonomicDrive.vi"("Rotation"=0.0, "Gyro Angle"=w1156, "Y"=0.0, "X"=0.0, "RobotDriveDevRef"=w1155) -> ()  [unwired: 4 in, 3 out]
        }
      }
    }
    frame "Three Totes" {
      n451 = call "WPI_SimpleGyro_RefNum Registry Get.vi"("refnum name"="SimpleGyro") -> ("error out"=w1207:errorcluster, "SimpleGyroDevRef"=w1211:T3)  [unwired: 9 in]
      n452 = call <vilib>:"WPI_RobotDriveRefNum Registry Get.vi"("refnum name"="Four Motors") -> ("error out"=w1206:errorcluster, "RobotDriveDevRef"=w1210:T6)  [unwired: 1 in, 8 out]
      n453 = call <vilib>:"WPI_EncoderRefNum Registry Get.vi"("refnum name"="Left Front Drive Encoder") -> ("error out"=w1205:errorcluster, "EncoderDevRef"=w1209:T15)  [unwired: 9 in]
      n454 = call <vilib>:"WPI_MotorControlRefNum Registry Get.vi"("refnum name"="ARI Motor") -> ("error out"=w1204:errorcluster, "MotorControlDevRef"=w1208:T7)  [unwired: 9 in]
      n455 = call <vilib>:"WPI_RelayRefNum Registry Get.vi"("refnum name"="Clamper Motor") -> ("error out"=w1201:errorcluster, "RelayDevRef"=w1202:T19)  [unwired: 9 in]
      n456 = call <vilib>:"WPI_MotorControlRefNum Registry Get.vi"("refnum name"="Lifter Motor") -> ("error out"=w1198:errorcluster, "MotorControlDevRef"=w1199:T7)  [unwired: 9 in]
      n457 = call <vilib>:"WPI_EncoderRefNum Registry Get.vi"("refnum name"="Lifter Motor Encoder") -> ("error out"=w1195:errorcluster, "EncoderDevRef"=w1196:T15)  [unwired: 9 in]
      n458 = Bundle("SimpleGyroDevRef"=w1211, "RobotDriveDevRef"=w1210, "EncoderDevRef"=w1209, "MotorControlDevRef"=w1208, "RelayDevRef"=w1202, "MotorControlDevRef"=w1199, "EncoderDevRef"=w1196) -> (w1194:T24)  [unwired: 1 in]
      n459 = Bundle("error out"=w1207, "error out"=w1206, "error out"=w1205, "error out"=w1204, "error out"=w1201, "error out"=w1198, "error out"=w1195) -> ()  [unwired: 1 in, 1 out]
      n460 = flat-sequence {
        tunnel: w1194 -> [w1221]
        tunnel: [w1221] -> w1218
        tunnel: w1218 -> [w1226]
        tunnel: [w1226] -> w1193
        tunnel: [w1225] -> w1171
        tunnel: [w1224] -> w1170
        tunnel: [w1258] -> w1217
        tunnel: w1193 -> [w1258]
        tunnel: w1171 -> [w1257]
        tunnel: w1170 -> [w1256]
        tunnel: w1217 -> [w1259]
        tunnel: [w1259] -> w1169
        tunnel: w1169 -> [w1289]
        tunnel: [w1289] -> w1168
        tunnel: [w1291] -> w1167
        tunnel: [w1290] -> w1166
        tunnel: w1168 -> [w1324]
        tunnel: [w1324] -> w1192
        tunnel: w1167 -> [w1327]
        tunnel: w1166 -> [w1326]
        tunnel: w1192 -> [w1329]
        tunnel: [w1329] -> w1191
        tunnel: [w1328] -> w1189
        tunnel: [w1341] -> w1216
        tunnel: w1191 -> [w1341]
        tunnel: w1189 -> [w1343]
        tunnel: w1216 -> [w1347]
        tunnel: [w1347] -> w1165
        tunnel: [w1346] -> w1163
        tunnel: [w1344] -> w1161
        tunnel: w1165 -> [w1382]
        tunnel: [w1382] -> w1164
        tunnel: w1163 -> [_]
        tunnel: [w1378] -> w1162
        tunnel: w1161 -> [_]
        tunnel: [w1379] -> w1160
        tunnel: w1164 -> [w1415]
        tunnel: [w1415] -> w1190
        tunnel: w1162 -> [w1414]
        tunnel: w1160 -> [w1413]
        tunnel: w1190 -> [w1417]
        tunnel: [w1417] -> w1188
        tunnel: [w1416] -> w1186
        tunnel: w1188 -> [w1429]
        tunnel: [w1429] -> w1187
        tunnel: w1186 -> [w1430]
        tunnel: w1187 -> [w1434]
        tunnel: [w1434] -> w1185
        tunnel: [w1433] -> w1183
        tunnel: [w1432] -> w1182
        tunnel: w1185 -> [w1469]
        tunnel: [w1469] -> w1184
        tunnel: w1183 -> [w1467]
        tunnel: w1182 -> [w1466]
        tunnel: w1184 -> [w1471]
        tunnel: [w1471] -> w1181
        tunnel: [w1470] -> w1180
        tunnel: w1181 -> [w1483]
        tunnel: w1180 -> [w1484]
        tunnel: [w1483] -> w1179
        tunnel: w1179 -> [w1488]
        tunnel: [w1488] -> w1178
        tunnel: [w1487] -> w1177
        tunnel: [w1486] -> w1176
        tunnel: w1178 -> [w1520]
        tunnel: [w1520] -> w1175
        tunnel: w1177 -> [w1518]
        tunnel: w1176 -> [w1517]
        tunnel: w1175 -> [w1522]
        tunnel: [w1522] -> w1174
        tunnel: [w1521] -> w1172
        tunnel: w1174 -> [w1536]
        tunnel: [w1536] -> w1173
        tunnel: w1172 -> [w1534]
        tunnel: [w1537] -> _
        tunnel: w1173 -> [w1537]
        frame #0 {
          n461 = Unbundle By Name(w1221) -> ("SimpleGyroDevRef"=w1222:T3, "EncoderDevRef"=w1223:T15, "EncoderDevRef"=w1220:T15)
          n462 = call "WPI_SimpleGyro_Reset.vi"("Reset? (T)"=TRUE, "SimpleGyroDevRef"=w1222) -> ()  [unwired: 8 in, 2 out]
          n463 = call <vilib>:"WPI_EncoderReset.vi"("EncoderDevRef"=w1223) -> ()  [unwired: 9 in, 2 out]
          n464 = call <vilib>:"WPI_EncoderReset.vi"("EncoderDevRef"=w1220) -> ()  [unwired: 9 in, 2 out]
        }
        frame #1 {
          # "Strafe left"
          n465 = Unbundle By Name(w1226) -> ("SimpleGyroDevRef"=w1227:T3, "RobotDriveDevRef"=w1229:T6, "EncoderDevRef"=w1228:T15)
          n466 = while {
            tunnel: w1229 -> [w1241]
            tunnel: w1228 -> [w1232]
            tunnel: [w1240] -> w1224
            tunnel: w1227 -> [w1236]
            tunnel: [w1233] -> w1225
            stop <- w1242 stop-if-true
            n467 = global read "Robot Global Data.vi" "Competition Robot?"() -> (w1244:bool)
            n468 = call "WPI_SimpleGyro_Get Angle.vi"("SimpleGyroDevRef"=w1236) -> ("Angle"=w1235:dbl)  [unwired: 8 in, 2 out]
            n469 = call <vilib>:"WPI_EncoderGet.vi"("EncoderDevRef"=w1232) -> ("Distance"=w1230:dbl, "EncoderDevRef"=w1240:T15)  [unwired: 5 in, 4 out]
            n470 = call-poly <vilib>:"SD Write Value.vi"("Numeric"=w1230, "Name"="Wheel Encoder") -> ()  [unwired: 8 in, 2 out]
            n471 = call-poly <vilib>:"PID.vi"("output range"=cluster{"output high":dbl, "output low":dbl} {"output high"=0.1, "output low"=-0.10000000000000003}, "PID gains"=T2 {"proportional gain (Kc)"=1.2, "integral time (Ti, min)"=0.2, "derivative time (Td, min)"=0.02}, "process variable"=w1235, "setpoint"=0.0) -> ("output"=w1234:dbl)  [unwired: 6 in, 1 out]
            n472 = case shown="True" w1244 {
              tunnel: w1241 -> [w1247 w1252]
              tunnel: w1234 -> [w1245 w1250]
              tunnel: [w1246 w1251] -> w1233
              frame True {
                n473 = call-poly <vilib>:"WPI_RobotDriveHolonomicDrive.vi"("Rotation"=w1245, "Y"=0.0 ("X axis value"), "X"=0.5 ("X axis value"), "RobotDriveDevRef"=w1247) -> ("RobotDriveDevRef"=w1246:T6)  [unwired: 5 in, 2 out]
              }
              frame False {
                n474 = call-poly <vilib>:"WPI_RobotDriveHolonomicDrive.vi"("Rotation"=w1250, "Y"=0.0 ("X axis value"), "X"=-0.5 ("X axis value"), "RobotDriveDevRef"=w1252) -> ("RobotDriveDevRef"=w1251:T6)  [unwired: 5 in, 2 out]
              }
            }
            n475 = Less Or Equal?(x=w1230, y=-500.0) -> (x <= y?=w1242:bool)
          }
        }
        frame #2 {
          w1255 = 0.0 ("X")
          n476 = call <vilib>:"WPI_EncoderReset.vi"("EncoderDevRef"=w1256) -> ()  [unwired: 9 in, 2 out]
          n477 = call-poly <vilib>:"WPI_RobotDriveHolonomicDrive.vi"("Rotation"=w1255, "Y"=w1255, "X"=w1255, "RobotDriveDevRef"=w1257) -> ()  [unwired: 5 in, 3 out]
        }
        frame #3 {
          # "Drive forward to tote #1"
          n478 = Unbundle By Name(w1259) -> ("SimpleGyroDevRef"=w1260:T3, "RobotDriveDevRef"=w1262:T6, "EncoderDevRef"=w1261:T15)
          n479 = while {
            tunnel: w1262 -> [w1270]
            tunnel: w1261 -> [w1269]
            tunnel: w1260 -> [w1266]
            stop <- w1271 stop-if-true
            n480 = global read "Robot Global Data.vi" "Competition Robot?"() -> (w1274:bool)
            n481 = call "WPI_SimpleGyro_Get Angle.vi"("SimpleGyroDevRef"=w1266) -> ("Angle"=w1265:dbl)  [unwired: 8 in, 2 out]
            n482 = call <vilib>:"WPI_EncoderGet.vi"("EncoderDevRef"=w1269) -> ("Distance"=w1273:dbl)  [unwired: 5 in, 5 out]
            n483 = call-poly <vilib>:"PID.vi"("output range"=cluster{"output high":dbl, "output low":dbl} {"output high"=0.1, "output low"=-0.1}, "PID gains"=T2 {"proportional gain (Kc)"=3.0, "integral time (Ti, min)"=0.002, "derivative time (Td, min)"=0.0}, "process variable"=w1265, "setpoint"=0.0) -> ("output"=w1263:dbl)  [unwired: 6 in, 1 out]
            n484 = case shown="False" w1274 {
              tunnel: w1270 -> [w1279 w1286]
              tunnel: w1263 -> [w1277 w1285]
              tunnel: [w1276 w1283] -> _
              frame True {
                n485 = Multiply(x=w1277, y=-1.0) -> (x*y=w1275:dbl)
                n486 = call-poly <vilib>:"WPI_RobotDriveHolonomicDrive.vi"("Rotation"=w1275, "Y"=0.28 ("X axis value"), "X"=0.0 ("X axis value"), "RobotDriveDevRef"=w1279) -> ("RobotDriveDevRef"=w1276:T6)  [unwired: 5 in, 2 out]
              }
              frame False {
                n487 = Multiply(x=w1285, y=1.0) -> (x*y=w1282:dbl)
                n488 = call-poly <vilib>:"WPI_RobotDriveHolonomicDrive.vi"("Rotation"=w1282, "Y"=-0.35 ("X axis value"), "X"=0.0 ("X axis value"), "RobotDriveDevRef"=w1286) -> ("RobotDriveDevRef"=w1283:T6)  [unwired: 5 in, 2 out]
              }
            }
            n489 = Greater Or Equal?(x=w1273, y=100.0) -> (x >= y?=w1271:bool)
          }
        }
        frame #4 {
          # "Drive forward to tote #1"
          n490 = Unbundle By Name(w1289) -> ("SimpleGyroDevRef"=w1292:T3, "RobotDriveDevRef"=w1294:T6, "EncoderDevRef"=w1293:T15)
          n491 = while {
            tunnel: w1294 -> [w1304]
            tunnel: w1293 -> [w1303]
            tunnel: [w1302] -> w1290
            tunnel: w1292 -> [w1299]
            tunnel: [w1295] -> w1291
            stop <- w1305 stop-if-true
            n492 = global read "Robot Global Data.vi" "Competition Robot?"() -> (w1308:bool)
            n493 = call "WPI_SimpleGyro_Get Angle.vi"("SimpleGyroDevRef"=w1299) -> ("Angle"=w1298:dbl)  [unwired: 8 in, 2 out]
            n494 = call <vilib>:"WPI_EncoderGet.vi"("EncoderDevRef"=w1303) -> ("Distance"=w1307:dbl, "EncoderDevRef"=w1302:T15)  [unwired: 5 in, 4 out]
            n495 = call-poly <vilib>:"PID.vi"("output range"=cluster{"output high":dbl, "output low":dbl} {"output high"=0.1, "output low"=-0.1}, "PID gains"=T2 {"proportional gain (Kc)"=3.0, "integral time (Ti, min)"=0.002, "derivative time (Td, min)"=0.0}, "process variable"=w1298, "setpoint"=0.0) -> ("output"=w1296:dbl)  [unwired: 6 in, 1 out]
            n496 = case shown="False" w1308 {
              tunnel: w1304 -> [w1313 w1320]
              tunnel: w1296 -> [w1311 w1319]
              tunnel: [w1310 w1317] -> w1295
              frame True {
                n497 = Multiply(x=w1311, y=-1.0) -> (x*y=w1309:dbl)
                n498 = call-poly <vilib>:"WPI_RobotDriveHolonomicDrive.vi"("Rotation"=w1309, "Y"=0.18 ("X axis value"), "X"=0.0 ("X axis value"), "RobotDriveDevRef"=w1313) -> ("RobotDriveDevRef"=w1310:T6)  [unwired: 5 in, 2 out]
              }
              frame False {
                n499 = Multiply(x=w1319, y=1.0) -> (x*y=w1316:dbl)
                n500 = call-poly <vilib>:"WPI_RobotDriveHolonomicDrive.vi"("Rotation"=w1316, "Y"=-0.1 ("X axis value"), "X"=0.0 ("X axis value"), "RobotDriveDevRef"=w1320) -> ("RobotDriveDevRef"=w1317:T6)  [unwired: 5 in, 2 out]
              }
            }
            n501 = Greater Or Equal?(x=w1307, y=185.0) -> (x >= y?=w1305:bool)
          }
        }
        frame #5 {
          w1323 = 0.0 ("X")
          n502 = Unbundle By Name(w1324) -> ("EncoderDevRef"=w1325:T15)
          n503 = call <vilib>:"WPI_EncoderReset.vi"("EncoderDevRef"=w1326) -> ()  [unwired: 9 in, 2 out]
          n504 = call-poly <vilib>:"WPI_RobotDriveHolonomicDrive.vi"("Rotation"=w1323, "Y"=w1323, "X"=w1323, "RobotDriveDevRef"=w1327) -> ()  [unwired: 5 in, 3 out]
          n505 = call <vilib>:"WPI_EncoderReset.vi"("EncoderDevRef"=w1325) -> ()  [unwired: 9 in, 2 out]
        }
        frame #6 {
          # "Pick up tote #1"
          n506 = while {
            tunnel: w1329 -> [w1332]
            tunnel: [w1330] -> w1328
            stop <- w1331 stop-if-true
            n507 = Unbundle By Name(w1332) -> ("MotorControlDevRef"=w1340:T7, "EncoderDevRef"=w1338:T15)
            n508 = call <vilib>:"WPI_EncoderGet.vi"("EncoderDevRef"=w1338) -> ("Distance"=w1337:dbl)  [unwired: 5 in, 5 out]
            n509 = call-poly <vilib>:"PID.vi"("output range"=cluster{"output high":dbl, "output low":dbl} {"output high"=1.0, "output low"=-1.0}, "PID gains"=T2 {"proportional gain (Kc)"=1.0, "integral time (Ti, min)"=0.001, "derivative time (Td, min)"=0.0}, "process variable"=w1337, "setpoint"=270.0) -> ("output"=w1336:dbl)  [unwired: 6 in, 1 out]
            n510 = Greater?(x=w1337, y=265.0) -> (0:w1331:bool)
            n511 = call <vilib>:"WPI_MotorControlSetOutput.vi"("Output"=w1336, "MotorControlDevRef"=w1340) -> ("MotorControlDevRef"=w1330:T7)  [unwired: 7 in, 2 out]
          }
        }
        frame #7 {
          n512 = call <vilib>:"WPI_MotorControlSetOutput.vi"("Output"=0.0, "MotorControlDevRef"=w1343) -> ()  [unwired: 7 in, 3 out]
        }
        frame #8 {
          # "Drive Forward to pick up tote #2"
          n513 = Unbundle By Name(w1347) -> ("SimpleGyroDevRef"=w1345:T3, "RobotDriveDevRef"=w1349:T6, "EncoderDevRef"=w1348:T15)
          n514 = while {
            tunnel: w1349 -> [w1359]
            tunnel: w1348 -> [w1358]
            tunnel: [w1357] -> w1346
            tunnel: w1345 -> [w1354]
            tunnel: [w1350] -> w1344
            stop <- w1360 stop-if-true
            n515 = global read "Robot Global Data.vi" "Competition Robot?"() -> (w1363:bool)
            n516 = call "WPI_SimpleGyro_Get Angle.vi"("SimpleGyroDevRef"=w1354) -> ("Angle"=w1353:dbl)  [unwired: 8 in, 2 out]
            n517 = call <vilib>:"WPI_EncoderGet.vi"("EncoderDevRef"=w1358) -> ("Distance"=w1362:dbl, "EncoderDevRef"=w1357:T15)  [unwired: 5 in, 4 out]
            n518 = call-poly <vilib>:"PID.vi"("output range"=cluster{"output high":dbl, "output low":dbl} {"output high"=0.15, "output low"=-0.15}, "PID gains"=T2 {"proportional gain (Kc)"=3.0, "integral time (Ti, min)"=0.002, "derivative time (Td, min)"=0.0}, "process variable"=w1353, "setpoint"=0.0) -> ("output"=w1351:dbl)  [unwired: 6 in, 1 out]
            n519 = case shown="False" w1363 {
              tunnel: w1359 -> [w1368 w1375]
              tunnel: w1351 -> [w1366 w1374]
              tunnel: [w1365 w1372] -> w1350
              frame True {
                n520 = Multiply(x=w1366, y=-1.0) -> (x*y=w1364:dbl)
                n521 = call-poly <vilib>:"WPI_RobotDriveHolonomicDrive.vi"("Rotation"=w1364, "Y"=0.28 ("X axis value"), "X"=0.0 ("X axis value"), "RobotDriveDevRef"=w1368) -> ("RobotDriveDevRef"=w1365:T6)  [unwired: 5 in, 2 out]
              }
              frame False {
                n522 = Multiply(x=w1374, y=1.02) -> (x*y=w1371:dbl)
                n523 = call-poly <vilib>:"WPI_RobotDriveHolonomicDrive.vi"("Rotation"=w1371, "Y"=-0.35 ("X axis value"), "X"=0.0 ("X axis value"), "RobotDriveDevRef"=w1375) -> ("RobotDriveDevRef"=w1372:T6)  [unwired: 5 in, 2 out]
              }
            }
            n524 = Greater Or Equal?(x=w1362, y=1140.0) -> (x >= y?=w1360:bool)
          }
        }
        frame #9 {
          # "Drive Forward to pick up tote  #2 SLOWLY"
          n525 = Unbundle By Name(w1382) -> ("SimpleGyroDevRef"=w1383:T3, "RobotDriveDevRef"=w1381:T6, "EncoderDevRef"=w1380:T15)
          n526 = while {
            tunnel: w1381 -> [w1393]
            tunnel: w1380 -> [w1392]
            tunnel: [w1391] -> w1378
            tunnel: w1383 -> [w1388]
            tunnel: [w1384] -> w1379
            stop <- w1394 stop-if-true
            n527 = global read "Robot Global Data.vi" "Competition Robot?"() -> (w1397:bool)
            n528 = call "WPI_SimpleGyro_Get Angle.vi"("SimpleGyroDevRef"=w1388) -> ("Angle"=w1387:dbl)  [unwired: 8 in, 2 out]
            n529 = call <vilib>:"WPI_EncoderGet.vi"("EncoderDevRef"=w1392) -> ("Distance"=w1396:dbl, "EncoderDevRef"=w1391:T15)  [unwired: 5 in, 4 out]
            n530 = call-poly <vilib>:"PID.vi"("output range"=cluster{"output high":dbl, "output low":dbl} {"output high"=0.15, "output low"=-0.15}, "PID gains"=T2 {"proportional gain (Kc)"=3.0, "integral time (Ti, min)"=0.002, "derivative time (Td, min)"=0.0}, "process variable"=w1387, "setpoint"=0.0) -> ("output"=w1385:dbl)  [unwired: 6 in, 1 out]
            n531 = case shown="False" w1397 {
              tunnel: w1393 -> [w1402 w1409]
              tunnel: w1385 -> [w1400 w1408]
              tunnel: [w1399 w1406] -> w1384
              frame True {
                n532 = Multiply(x=w1400, y=-1.0) -> (x*y=w1398:dbl)
                n533 = call-poly <vilib>:"WPI_RobotDriveHolonomicDrive.vi"("Rotation"=w1398, "Y"=0.28 ("X axis value"), "X"=0.0 ("X axis value"), "RobotDriveDevRef"=w1402) -> ("RobotDriveDevRef"=w1399:T6)  [unwired: 5 in, 2 out]
              }
              frame False {
                n534 = Multiply(x=w1408, y=1.018) -> (x*y=w1405:dbl)
                n535 = call-poly <vilib>:"WPI_RobotDriveHolonomicDrive.vi"("Rotation"=w1405, "Y"=-0.15 ("X axis value"), "X"=0.0 ("X axis value"), "RobotDriveDevRef"=w1409) -> ("RobotDriveDevRef"=w1406:T6)  [unwired: 5 in, 2 out]
              }
            }
            n536 = Greater Or Equal?(x=w1396, y=1540.0) -> (x >= y?=w1394:bool)
          }
        }
        frame #10 {
          w1412 = 0.0 ("X")
          n537 = call <vilib>:"WPI_EncoderReset.vi"("EncoderDevRef"=w1414) -> ()  [unwired: 9 in, 2 out]
          n538 = call-poly <vilib>:"WPI_RobotDriveHolonomicDrive.vi"("Rotation"=w1412, "Y"=w1412, "X"=w1412, "RobotDriveDevRef"=w1413) -> ()  [unwired: 5 in, 3 out]
        }
        frame #11 {
          # "Pick up tote #2"
          n539 = while {
            tunnel: w1417 -> [w1420]
            tunnel: [w1418] -> w1416
            stop <- w1419 stop-if-true
            n540 = Unbundle By Name(w1420) -> ("MotorControlDevRef"=w1428:T7, "EncoderDevRef"=w1426:T15)
            n541 = call <vilib>:"WPI_EncoderGet.vi"("EncoderDevRef"=w1426) -> ("Distance"=w1425:dbl)  [unwired: 5 in, 5 out]
            n542 = call-poly <vilib>:"PID.vi"("output range"=cluster{"output high":dbl, "output low":dbl} {"output high"=1.0, "output low"=-1.0}, "PID gains"=T2 {"proportional gain (Kc)"=3.0, "integral time (Ti, min)"=0.001, "derivative time (Td, min)"=0.0}, "process variable"=w1425, "setpoint"=510.0) -> ("output"=w1424:dbl)  [unwired: 6 in, 1 out]
            n543 = Greater?(x=w1425, y=510.0) -> (0:w1419:bool)
            n544 = call <vilib>:"WPI_MotorControlSetOutput.vi"("Output"=w1424, "MotorControlDevRef"=w1428) -> ("MotorControlDevRef"=w1418:T7)  [unwired: 7 in, 2 out]
          }
        }
        frame #12 {
          n545 = call <vilib>:"WPI_MotorControlSetOutput.vi"("Output"=0.0, "MotorControlDevRef"=w1430) -> ()  [unwired: 7 in, 3 out]
        }
        frame #13 {
          # "Drive forward to tote #3"
          n546 = Unbundle By Name(w1434) -> ("SimpleGyroDevRef"=w1435:T3, "RobotDriveDevRef"=w1437:T6, "EncoderDevRef"=w1436:T15)
          n547 = while {
            tunnel: w1437 -> [w1447]
            tunnel: w1436 -> [w1446]
            tunnel: [w1445] -> w1433
            tunnel: w1435 -> [w1442]
            tunnel: [w1438] -> w1432
            stop <- w1448 stop-if-true
            n548 = global read "Robot Global Data.vi" "Competition Robot?"() -> (w1451:bool)
            n549 = call "WPI_SimpleGyro_Get Angle.vi"("SimpleGyroDevRef"=w1442) -> ("Angle"=w1441:dbl)  [unwired: 8 in, 2 out]
            n550 = call <vilib>:"WPI_EncoderGet.vi"("EncoderDevRef"=w1446) -> ("Distance"=w1450:dbl, "EncoderDevRef"=w1445:T15)  [unwired: 5 in, 4 out]
            n551 = call-poly <vilib>:"PID.vi"("output range"=cluster{"output high":dbl, "output low":dbl} {"output high"=0.1, "output low"=-0.1}, "PID gains"=T2 {"proportional gain (Kc)"=1.0, "integral time (Ti, min)"=0.002, "derivative time (Td, min)"=0.0}, "process variable"=w1441, "setpoint"=0.0) -> ("output"=w1439:dbl)  [unwired: 6 in, 1 out]
            n552 = case shown="False" w1451 {
              tunnel: w1447 -> [w1456 w1463]
              tunnel: w1439 -> [w1454 w1462]
              tunnel: [w1453 w1460] -> w1438
              frame True {
                n553 = Multiply(x=w1454, y=-1.0) -> (x*y=w1452:dbl)
                n554 = call-poly <vilib>:"WPI_RobotDriveHolonomicDrive.vi"("Rotation"=w1452, "Y"=0.28 ("X axis value"), "X"=0.0 ("X axis value"), "RobotDriveDevRef"=w1456) -> ("RobotDriveDevRef"=w1453:T6)  [unwired: 5 in, 2 out]
              }
              frame False {
                n555 = Multiply(x=w1462, y=1.0) -> (x*y=w1459:dbl)
                n556 = call-poly <vilib>:"WPI_RobotDriveHolonomicDrive.vi"("Rotation"=w1459, "Y"=-0.35 ("X axis value"), "X"=0.0 ("X axis value"), "RobotDriveDevRef"=w1463) -> ("RobotDriveDevRef"=w1460:T6)  [unwired: 5 in, 2 out]
              }
            }
            n557 = Greater Or Equal?(x=w1450, y=1600.0) -> (x >= y?=w1448:bool)
          }
        }
        frame #14 {
          w1468 = 0.0 ("X")
          n558 = call <vilib>:"WPI_EncoderReset.vi"("EncoderDevRef"=w1467) -> ()  [unwired: 9 in, 2 out]
          n559 = call-poly <vilib>:"WPI_RobotDriveHolonomicDrive.vi"("Rotation"=w1468, "Y"=w1468, "X"=w1468, "RobotDriveDevRef"=w1466) -> ()  [unwired: 5 in, 3 out]
        }
        frame #15 {
          # "Pick up tote #3"
          n560 = while {
            tunnel: w1471 -> [w1474]
            tunnel: [w1472] -> w1470
            stop <- w1473 stop-if-true
            n561 = Unbundle By Name(w1474) -> ("MotorControlDevRef"=w1482:T7, "EncoderDevRef"=w1480:T15)
            n562 = call <vilib>:"WPI_EncoderGet.vi"("EncoderDevRef"=w1480) -> ("Distance"=w1479:dbl)  [unwired: 5 in, 5 out]
            n563 = call-poly <vilib>:"PID.vi"("output range"=cluster{"output high":dbl, "output low":dbl} {"output high"=1.0, "output low"=-1.0}, "PID gains"=T2 {"proportional gain (Kc)"=3.0, "integral time (Ti, min)"=0.0, "derivative time (Td, min)"=0.0}, "process variable"=w1479, "setpoint"=750.0) -> ("output"=w1478:dbl)  [unwired: 6 in, 1 out]
            n564 = Greater?(x=w1479, y=745.0) -> (0:w1473:bool)
            n565 = call <vilib>:"WPI_MotorControlSetOutput.vi"("Output"=w1478, "MotorControlDevRef"=w1482) -> ("MotorControlDevRef"=w1472:T7)  [unwired: 7 in, 2 out]
          }
        }
        frame #16 {
          n566 = call <vilib>:"WPI_MotorControlSetOutput.vi"("Output"=0.0, "MotorControlDevRef"=w1484) -> ()  [unwired: 7 in, 3 out]
        }
        frame #17 {
          # "Strafe right"
          n567 = Unbundle By Name(w1488) -> ("SimpleGyroDevRef"=w1489:T3, "RobotDriveDevRef"=w1491:T6, "EncoderDevRef"=w1490:T15)
          n568 = while {
            tunnel: w1491 -> [w1503]
            tunnel: w1490 -> [w1494]
            tunnel: [w1502] -> w1486
            tunnel: w1489 -> [w1498]
            tunnel: [w1495] -> w1487
            stop <- w1504 stop-if-true
            n569 = global read "Robot Global Data.vi" "Competition Robot?"() -> (w1506:bool)
            n570 = call "WPI_SimpleGyro_Get Angle.vi"("SimpleGyroDevRef"=w1498) -> ("Angle"=w1497:dbl)  [unwired: 8 in, 2 out]
            n571 = call <vilib>:"WPI_EncoderGet.vi"("EncoderDevRef"=w1494) -> ("Distance"=w1492:dbl, "EncoderDevRef"=w1502:T15)  [unwired: 5 in, 4 out]
            n572 = call-poly <vilib>:"SD Write Value.vi"("Numeric"=w1492, "Name"="Wheel Encoder") -> ()  [unwired: 8 in, 2 out]
            n573 = call-poly <vilib>:"PID.vi"("output range"=cluster{"output high":dbl, "output low":dbl} {"output high"=0.2, "output low"=-0.2}, "PID gains"=T2 {"proportional gain (Kc)"=1.2, "integral time (Ti, min)"=0.2, "derivative time (Td, min)"=0.02}, "process variable"=w1497, "setpoint"=0.0) -> ("output"=w1496:dbl)  [unwired: 6 in, 1 out]
            n574 = case shown="False" w1506 {
              tunnel: w1503 -> [w1509 w1514]
              tunnel: w1496 -> [w1507 w1512]
              tunnel: [w1508 w1513] -> w1495
              frame True {
                n575 = call-poly <vilib>:"WPI_RobotDriveHolonomicDrive.vi"("Rotation"=w1507, "Y"=0.0 ("X axis value"), "X"=-0.5 ("X axis value"), "RobotDriveDevRef"=w1509) -> ("RobotDriveDevRef"=w1508:T6)  [unwired: 5 in, 2 out]
              }
              frame False {
                n576 = call-poly <vilib>:"WPI_RobotDriveHolonomicDrive.vi"("Rotation"=w1512, "Y"=0.0 ("X axis value"), "X"=0.5 ("X axis value"), "RobotDriveDevRef"=w1514) -> ("RobotDriveDevRef"=w1513:T6)  [unwired: 5 in, 2 out]
              }
            }
            n577 = Greater Or Equal?(x=w1492, y=1800.0) -> (x >= y?=w1504:bool)
          }
        }
        frame #18 {
          w1519 = 0.0 ("X")
          n578 = call <vilib>:"WPI_EncoderReset.vi"("EncoderDevRef"=w1517) -> ()  [unwired: 9 in, 2 out]
          n579 = call-poly <vilib>:"WPI_RobotDriveHolonomicDrive.vi"("Rotation"=w1519, "Y"=w1519, "X"=w1519, "RobotDriveDevRef"=w1518) -> ()  [unwired: 5 in, 3 out]
        }
        frame #19 {
          # "Drops"
          n580 = while {
            tunnel: w1522 -> [w1533]
            tunnel: [w1531] -> w1521
            stop <- w1529 stop-if-true
            n581 = Unbundle By Name(w1533) -> ("MotorControlDevRef"=w1532:T7, "EncoderDevRef"=w1528:T15)
            n582 = call <vilib>:"WPI_EncoderGet.vi"("EncoderDevRef"=w1528) -> ("Distance"=w1527:dbl)  [unwired: 5 in, 5 out]
            n583 = call-poly <vilib>:"PID.vi"("output range"=cluster{"output high":dbl, "output low":dbl} {"output high"=1.0, "output low"=-1.0}, "PID gains"=T2 {"proportional gain (Kc)"=1.0, "integral time (Ti, min)"=0.001, "derivative time (Td, min)"=0.0}, "process variable"=w1527, "setpoint"=-750.0) -> ("output"=w1526:dbl)  [unwired: 6 in, 1 out]
            n584 = Less?(x=w1527, y=-155.0) -> (x < y?=w1529:bool)
            n585 = call <vilib>:"WPI_MotorControlSetOutput.vi"("Output"=w1526, "MotorControlDevRef"=w1532) -> ("MotorControlDevRef"=w1531:T7)  [unwired: 7 in, 2 out]
          }
        }
        frame #20 {
          n586 = call <vilib>:"WPI_MotorControlSetOutput.vi"("Output"=0.0, "MotorControlDevRef"=w1534) -> ()  [unwired: 7 in, 3 out]
        }
        frame #21 {
          n587 = Unbundle By Name(w1537) -> ("SimpleGyroDevRef"=w1538:T3, "RobotDriveDevRef"=w1539:T6)
          n588 = call "WPI_SimpleGyro_Get Angle.vi"("SimpleGyroDevRef"=w1538) -> ("Angle"=w1540:dbl)  [unwired: 8 in, 2 out]
          n589 = call-poly <vilib>:"WPI_RobotDriveHolonomicDrive.vi"("Rotation"=0.0, "Gyro Angle"=w1540, "Y"=0.0, "X"=0.0, "RobotDriveDevRef"=w1539) -> ()  [unwired: 4 in, 3 out]
        }
      }
    }
    frame "Dragon Tail" {
      n590 = call "WPI_SimpleGyro_RefNum Registry Get.vi"("refnum name"="SimpleGyro") -> ("error out"=w1581:errorcluster, "SimpleGyroDevRef"=w1585:T3)  [unwired: 9 in]
      n591 = call <vilib>:"WPI_RobotDriveRefNum Registry Get.vi"("refnum name"="Four Motors") -> ("error out"=w1580:errorcluster, "RobotDriveDevRef"=w1584:T6)  [unwired: 1 in, 8 out]
      n592 = call <vilib>:"WPI_EncoderRefNum Registry Get.vi"("refnum name"="Left Front Drive Encoder") -> ("error out"=w1579:errorcluster, "EncoderDevRef"=w1583:T15)  [unwired: 9 in]
      n593 = call <vilib>:"WPI_MotorControlRefNum Registry Get.vi"("refnum name"="ARI Motor") -> ("error out"=w1578:errorcluster, "MotorControlDevRef"=w1582:T7)  [unwired: 9 in]
      n594 = call <vilib>:"WPI_RelayRefNum Registry Get.vi"("refnum name"="Clamper Motor") -> ("error out"=w1575:errorcluster, "RelayDevRef"=w1576:T19)  [unwired: 9 in]
      n595 = call <vilib>:"WPI_RelayRefNum Registry Get.vi"("refnum name"="Lower Dragon Tail") -> ("error out"=w1563:errorcluster, "RelayDevRef"=w1565:T19)  [unwired: 9 in]
      n596 = call <vilib>:"WPI_MotorControlRefNum Registry Get.vi"("refnum name"="Lifter Motor") -> ("error out"=w1572:errorcluster, "MotorControlDevRef"=w1573:T7)  [unwired: 9 in]
      n597 = call <vilib>:"WPI_EncoderRefNum Registry Get.vi"("refnum name"="Lifter Motor Encoder") -> ("error out"=w1569:errorcluster, "EncoderDevRef"=w1570:T15)  [unwired: 9 in]
      n598 = call <vilib>:"WPI_RelayRefNum Registry Get.vi"("refnum name"="Extend Wings") -> ("error out"=w1564:errorcluster, "RelayDevRef"=w1566:T19)  [unwired: 9 in]
      n599 = Bundle("SimpleGyroDevRef"=w1585, "RobotDriveDevRef"=w1584, "EncoderDevRef"=w1583, "MotorControlDevRef"=w1582, "RelayDevRef"=w1576, "MotorControlDevRef"=w1573, "EncoderDevRef"=w1570, "RelayDevRef"=w1566, "RelayDevRef"=w1565) -> (w1562:T25)  [unwired: 1 in]
      n600 = Bundle("error out"=w1581, "error out"=w1580, "error out"=w1579, "error out"=w1578, "error out"=w1575, "error out"=w1572, "error out"=w1569, "error out"=w1564, "error out"=w1563) -> ()  [unwired: 1 in, 1 out]
      n601 = flat-sequence {
        tunnel: w1562 -> [w1590]
        tunnel: [w1590] -> w1561
        tunnel: w1561 -> [w1597]
        tunnel: [w1597] -> w1560
        tunnel: [w1596] -> w1559
        tunnel: [w1595] -> w1558
        tunnel: w1560 -> [w1607]
        tunnel: w1559 -> [w1606]
        tunnel: w1558 -> [w1605]
        tunnel: [w1607] -> w1557
        tunnel: w1557 -> [w1610]
        tunnel: [w1610] -> w1556
        tunnel: [w1609] -> w1555
        tunnel: [w1608] -> w1554
        tunnel: w1556 -> [w1620]
        tunnel: w1555 -> [w1618]
        tunnel: w1554 -> [w1617]
        tunnel: [w1620] -> w1553
        tunnel: w1553 -> [w1623]
        tunnel: [w1623] -> w1552
        tunnel: [w1622] -> w1551
        tunnel: [w1621] -> w1550
        tunnel: w1552 -> [w1633]
        tunnel: w1551 -> [w1631]
        tunnel: w1550 -> [w1630]
        tunnel: [w1633] -> w1549
        tunnel: w1549 -> [w1636]
        tunnel: [w1636] -> w1548
        tunnel: [w1635] -> w1547
        tunnel: [w1634] -> w1546
        tunnel: w1548 -> [w1646]
        tunnel: w1547 -> [w1644]
        tunnel: w1546 -> [w1643]
        tunnel: [w1646] -> w1545
        tunnel: w1545 -> [w1648]
        tunnel: [w1647] -> w1544
        tunnel: [w1674] -> _
        tunnel: w1544 -> [w1674]
        frame #0 {
          n602 = Unbundle By Name(w1590) -> ("SimpleGyroDevRef"=w1593:T3, "EncoderDevRef"=w1594:T15, "EncoderDevRef"=w1592:T15)
          n603 = call "WPI_SimpleGyro_Reset.vi"("Reset? (T)"=TRUE, "SimpleGyroDevRef"=w1593) -> ()  [unwired: 8 in, 2 out]
          n604 = call <vilib>:"WPI_EncoderReset.vi"("EncoderDevRef"=w1594) -> ()  [unwired: 9 in, 2 out]
          n605 = call <vilib>:"WPI_EncoderReset.vi"("EncoderDevRef"=w1592) -> ()  [unwired: 9 in, 2 out]
        }
        frame #1 {
          # "Lower halfway"
          n606 = while {
            tunnel: w1597 -> [w1603]
            tunnel: [w1599] -> w1596
            tunnel: [w1598] -> w1595
            stop <- w1600 stop-if-true
            n607 = Unbundle By Name(w1603) -> ("RelayDevRef"=w1602:T19)
            n608 = call "Clamper Time6"() -> ("Time has Elapsed"=w1600:bool)  [unwired: 12 in, 7 out]
            n609 = call <vilib>:"WPI_RelaySet.vi"("RelayValue"=WPI_RelayValue."Forward", "RelayDevRef"=w1602) -> ("error out"=w1598:errorcluster, "RelayDevRef"=w1599:T19)  [unwired: 8 in]
          }
        }
        frame #2 {
          n610 = call <vilib>:"WPI_RelaySet.vi"("error in (no error)"=w1605, "RelayValue"=WPI_RelayValue."Off", "RelayDevRef"=w1606) -> ()  [unwired: 7 in, 2 out]
        }
        frame #3 {
          # "Open wings"
          n611 = while {
            tunnel: w1610 -> [w1616]
            tunnel: [w1612] -> w1608
            tunnel: [w1611] -> w1609
            stop <- w1613 stop-if-true
            n612 = Unbundle By Name(w1616) -> ("RelayDevRef"=w1615:T19)
            n613 = call "Clamper Time7"() -> ("Time has Elapsed"=w1613:bool)  [unwired: 12 in, 7 out]
            n614 = call <vilib>:"WPI_RelaySet.vi"("RelayValue"=WPI_RelayValue."Forward", "RelayDevRef"=w1615) -> ("error out"=w1611:errorcluster, "RelayDevRef"=w1612:T19)  [unwired: 8 in]
          }
        }
        frame #4 {
          n615 = call <vilib>:"WPI_RelaySet.vi"("error in (no error)"=w1618, "RelayValue"=WPI_RelayValue."Off", "RelayDevRef"=w1617) -> ()  [unwired: 7 in, 2 out]
        }
        frame #5 {
          # "Lower all the way"
          n616 = while {
            tunnel: w1623 -> [w1629]
            tunnel: [w1625] -> w1622
            tunnel: [w1624] -> w1621
            stop <- w1626 stop-if-true
            n617 = Unbundle By Name(w1629) -> ("RelayDevRef"=w1628:T19)
            n618 = call "Clamper Time8"() -> ("Time has Elapsed"=w1626:bool)  [unwired: 12 in, 7 out]
            n619 = call <vilib>:"WPI_RelaySet.vi"("RelayValue"=WPI_RelayValue."Forward", "RelayDevRef"=w1628) -> ("error out"=w1624:errorcluster, "RelayDevRef"=w1625:T19)  [unwired: 8 in]
          }
        }
        frame #6 {
          n620 = call <vilib>:"WPI_RelaySet.vi"("error in (no error)"=w1630, "RelayValue"=WPI_RelayValue."Off", "RelayDevRef"=w1631) -> ()  [unwired: 7 in, 2 out]
        }
        frame #7 {
          # "Close wings"
          n621 = while {
            tunnel: w1636 -> [w1642]
            tunnel: [w1638] -> w1635
            tunnel: [w1637] -> w1634
            stop <- w1639 stop-if-true
            n622 = Unbundle By Name(w1642) -> ("RelayDevRef"=w1641:T19)
            n623 = call "Clamper Time9"() -> ("Time has Elapsed"=w1639:bool)  [unwired: 12 in, 7 out]
            n624 = call <vilib>:"WPI_RelaySet.vi"("RelayValue"=WPI_RelayValue."Forward", "RelayDevRef"=w1641) -> ("error out"=w1637:errorcluster, "RelayDevRef"=w1638:T19)  [unwired: 8 in]
          }
        }
        frame #8 {
          n625 = call <vilib>:"WPI_RelaySet.vi"("error in (no error)"=w1643, "RelayValue"=WPI_RelayValue."Off", "RelayDevRef"=w1644) -> ()  [unwired: 7 in, 2 out]
        }
        frame #9 {
          # "Drive backward to auto zone"
          n626 = while {
            tunnel: w1648 -> [w1652]
            tunnel: [w1652] -> w1647
            stop <- w1653 stop-if-true
            n627 = Unbundle By Name(w1652) -> ("SimpleGyroDevRef"=w1651:T3, "RobotDriveDevRef"=w1650:T6, "EncoderDevRef"=w1649:T15)
            n628 = global read "Robot Global Data.vi" "Competition Robot?"() -> (w1661:bool)
            n629 = call "WPI_SimpleGyro_Get Angle.vi"("SimpleGyroDevRef"=w1651) -> ("Angle"=w1656:dbl)  [unwired: 8 in, 2 out]
            n630 = call <vilib>:"WPI_EncoderGet.vi"("EncoderDevRef"=w1649) -> ("Distance"=w1660:dbl)  [unwired: 5 in, 5 out]
            n631 = call-poly <vilib>:"PID.vi"("output range"=cluster{"output high":dbl, "output low":dbl} {"output high"=0.1, "output low"=-0.1}, "PID gains"=T2 {"proportional gain (Kc)"=1.0, "integral time (Ti, min)"=0.002, "derivative time (Td, min)"=0.0}, "process variable"=w1656, "setpoint"=0.0) -> ("output"=w1654:dbl)  [unwired: 6 in, 1 out]
            n632 = case shown="False" w1661 {
              tunnel: w1650 -> [w1666 w1671]
              tunnel: w1654 -> [w1664 w1669]
              tunnel: [w1663 w1670] -> _
              frame True {
                n633 = Multiply(x=w1664, y=-1.0) -> (x*y=w1662:dbl)
                n634 = call-poly <vilib>:"WPI_RobotDriveHolonomicDrive.vi"("Rotation"=w1662, "Y"=-0.28 ("X axis value"), "X"=0.0 ("X axis value"), "RobotDriveDevRef"=w1666) -> ("RobotDriveDevRef"=w1663:T6)  [unwired: 5 in, 2 out]
              }
              frame False {
                n635 = call-poly <vilib>:"WPI_RobotDriveHolonomicDrive.vi"("Rotation"=w1669, "Y"=0.35 ("X axis value"), "X"=0.0 ("X axis value"), "RobotDriveDevRef"=w1671) -> ("RobotDriveDevRef"=w1670:T6)  [unwired: 5 in, 2 out]
              }
            }
            n636 = Greater Or Equal?(x=w1660, y=-800.0) -> (x >= y?=w1653:bool)
          }
        }
        frame #10 {
          n637 = Unbundle By Name(w1674) -> ("SimpleGyroDevRef"=w1675:T3, "RobotDriveDevRef"=w1676:T6)
          n638 = call "WPI_SimpleGyro_Get Angle.vi"("SimpleGyroDevRef"=w1675) -> ("Angle"=w1677:dbl)  [unwired: 8 in, 2 out]
          n639 = call-poly <vilib>:"WPI_RobotDriveHolonomicDrive.vi"("Rotation"=0.0, "Gyro Angle"=w1677, "Y"=0.0, "X"=0.0, "RobotDriveDevRef"=w1676) -> ()  [unwired: 4 in, 3 out]
        }
      }
    }
    frame "Can Left" {
      n640 = call "WPI_SimpleGyro_RefNum Registry Get.vi"("refnum name"="SimpleGyro") -> ("error out"=w1696:errorcluster, "SimpleGyroDevRef"=w1700:T3)  [unwired: 9 in]
      n641 = call <vilib>:"WPI_RobotDriveRefNum Registry Get.vi"("refnum name"="Four Motors") -> ("error out"=w1695:errorcluster, "RobotDriveDevRef"=w1699:T6)  [unwired: 1 in, 8 out]
      n642 = call <vilib>:"WPI_EncoderRefNum Registry Get.vi"("refnum name"="Left Front Drive Encoder") -> ("error out"=w1694:errorcluster, "EncoderDevRef"=w1698:T15)  [unwired: 9 in]
      n643 = call <vilib>:"WPI_MotorControlRefNum Registry Get.vi"("refnum name"="ARI Motor") -> ("error out"=w1693:errorcluster, "MotorControlDevRef"=w1697:T7)  [unwired: 9 in]
      n644 = call <vilib>:"WPI_RelayRefNum Registry Get.vi"("refnum name"="Clamper Motor") -> ("error out"=w1690:errorcluster, "RelayDevRef"=w1691:T19)  [unwired: 9 in]
      n645 = Bundle("SimpleGyroDevRef"=w1700, "RobotDriveDevRef"=w1699, "EncoderDevRef"=w1698, "MotorControlDevRef"=w1697, "RelayDevRef"=w1691) -> (w1685:T22)  [unwired: 1 in]
      n646 = Bundle("error out"=w1696, "error out"=w1695, "error out"=w1694, "error out"=w1693, "error out"=w1690) -> ()  [unwired: 1 in, 1 out]
      n647 = flat-sequence {
        tunnel: [w1712] -> w1686
        tunnel: w1685 -> [w1712]
        tunnel: [w1717] -> w1710
        tunnel: [w1716] -> w1709
        tunnel: [w1715] -> w1687
        tunnel: w1686 -> [w1715]
        tunnel: w1710 -> [w1725]
        tunnel: w1709 -> [w1724]
        tunnel: [w1723] -> w1688
        tunnel: w1687 -> [w1723]
        tunnel: [w1730] -> w1708
        tunnel: [w1729] -> w1707
        tunnel: [w1728] -> w1689
        tunnel: w1688 -> [w1728]
        tunnel: w1708 -> [w1738]
        tunnel: w1707 -> [w1737]
        tunnel: w1689 -> [w1736]
        tunnel: [w1736] -> w1684
        tunnel: [w1743] -> w1706
        tunnel: [w1742] -> w1705
        tunnel: w1684 -> [w1741]
        tunnel: [w1740] -> w1682
        tunnel: w1706 -> [w1768]
        tunnel: w1705 -> [w1767]
        tunnel: [w1766] -> w1683
        tunnel: w1682 -> [w1766]
        tunnel: w1683 -> [w1770]
        tunnel: [w1769] -> w1681
        tunnel: w1681 -> [w1791]
        frame #0 {
          n648 = Unbundle By Name(w1712) -> ("SimpleGyroDevRef"=w1713:T3, "EncoderDevRef"=w1711:T15)
          n649 = call "WPI_SimpleGyro_Reset.vi"("SimpleGyroDevRef"=w1713) -> ()  [unwired: 9 in, 2 out]
          n650 = call <vilib>:"WPI_EncoderReset.vi"("EncoderDevRef"=w1711) -> ()  [unwired: 9 in, 2 out]
        }
        frame #1 {
          n651 = Unbundle By Name(w1715) -> ("RelayDevRef"=w1714:T19)
          n652 = while {
            tunnel: [w1721] -> w1717
            tunnel: [w1720] -> w1716
            tunnel: w1714 -> [w1718]
            stop <- w1719 stop-if-true
            n653 = call "Clamper Time3"() -> ("Time has Elapsed"=w1719:bool)  [unwired: 12 in, 7 out]
            n654 = call <vilib>:"WPI_RelaySet.vi"("RelayValue"=WPI_RelayValue."Forward", "RelayDevRef"=w1718) -> ("error out"=w1720:errorcluster, "RelayDevRef"=w1721:T19)  [unwired: 8 in]
          }
        }
        frame #2 {
          n655 = call <vilib>:"WPI_RelaySet.vi"("error in (no error)"=w1724, "RelayValue"=WPI_RelayValue."Off", "RelayDevRef"=w1725) -> ()  [unwired: 7 in, 2 out]
        }
        frame #3 {
          n656 = Unbundle By Name(w1728) -> ("MotorControlDevRef"=w1727:T7)
          n657 = while {
            tunnel: [w1733] -> w1730
            tunnel: [w1732] -> w1729
            tunnel: w1727 -> [w1731]
            stop <- w1735 stop-if-true
            n658 = call "ARI Time3"() -> ("Time has Elapsed"=w1735:bool)  [unwired: 12 in, 7 out]
            n659 = call <vilib>:"WPI_MotorControlSetOutput.vi"("Output"=1.0, "MotorControlDevRef"=w1731) -> ("error out"=w1733:errorcluster, "MotorControlDevRef"=w1732:T7)  [unwired: 7 in, 1 out]
          }
        }
        frame #4 {
          n660 = call <vilib>:"WPI_MotorControlSetOutput.vi"("error in (no error)"=w1738, "Output"=0.0, "MotorControlDevRef"=w1737) -> ()  [unwired: 6 in, 3 out]
        }
        frame #5 {
          n661 = while {
            tunnel: [w1752] -> w1743
            tunnel: [w1751] -> w1742
            tunnel: w1741 -> [w1747]
            tunnel: [w1747] -> w1740
            stop <- w1753 stop-if-true
            n662 = Unbundle By Name(w1747) -> ("EncoderDevRef"=w1746:T15, "SimpleGyroDevRef"=w1745:T3, "RobotDriveDevRef"=w1744:T6)
            n663 = Wait (ms)(milliseconds to wait=u32 30) -> ()  [unwired: 1 out]
            n664 = global read "Robot Global Data.vi" "Competition Robot?"() -> (w1749:bool)
            n665 = call <vilib>:"WPI_EncoderGet.vi"("EncoderDevRef"=w1746) -> ("error out"=w1751:errorcluster, "Distance"=w1755:dbl, "EncoderDevRef"=w1752:T15)  [unwired: 5 in, 3 out]
            n666 = Greater Or Equal?(x=w1755, y=1660.0) -> (x >= y?=w1753:bool)
            n667 = call "WPI_SimpleGyro_Get Angle.vi"("SimpleGyroDevRef"=w1745) -> ("Angle"=w1750:dbl)  [unwired: 8 in, 2 out]
            n668 = case shown="False" w1749 {
              tunnel: w1750 -> [w1757 w1762]
              tunnel: w1744 -> [w1756 w1761]
              frame True {
                n669 = call-poly <vilib>:"WPI_RobotDriveHolonomicDrive.vi"("Rotation"=0.0, "Gyro Angle"=w1757, "Y"=0.4 ("X axis value"), "X"=0.0 ("X axis value"), "RobotDriveDevRef"=w1756) -> ()  [unwired: 4 in, 3 out]
              }
              frame False {
                n670 = call-poly <vilib>:"WPI_RobotDriveHolonomicDrive.vi"("Rotation"=0.0, "Gyro Angle"=w1762, "Y"=-0.4 ("X axis value"), "X"=0.0 ("X axis value"), "RobotDriveDevRef"=w1761) -> ()  [unwired: 4 in, 3 out]
              }
            }
          }
        }
        frame #6 {
          n671 = call <vilib>:"WPI_EncoderReset.vi"("error in (no error)"=w1767, "EncoderDevRef"=w1768) -> ()  [unwired: 8 in, 2 out]
        }
        frame #7 {
          n672 = while {
            tunnel: w1770 -> [w1773]
            tunnel: [w1773] -> w1769
            stop <- w1775 stop-if-true
            n673 = Unbundle By Name(w1773) -> ("SimpleGyroDevRef"=w1772:T3, "RobotDriveDevRef"=w1771:T6)
            n674 = global read "Robot Global Data.vi" "Competition Robot?"() -> (w1777:bool)
            n675 = Wait (ms)(milliseconds to wait=u32 30) -> ()  [unwired: 1 out]
            n676 = call "WPI_SimpleGyro_Get Angle.vi"("SimpleGyroDevRef"=w1772) -> ("Angle"=w1776:dbl)  [unwired: 8 in, 2 out]
            n677 = case shown="True" w1777 {
              tunnel: w1776 -> [w1780 w1785]
              tunnel: w1771 -> [w1779 w1784]
              frame True {
                n678 = call-poly <vilib>:"WPI_RobotDriveHolonomicDrive.vi"("Rotation"=0.25, "Gyro Angle"=w1780, "Y"=0.0 ("X axis value"), "X"=0.0 ("X axis value"), "RobotDriveDevRef"=w1779) -> ()  [unwired: 4 in, 3 out]
              }
              frame False {
                n679 = call-poly <vilib>:"WPI_RobotDriveHolonomicDrive.vi"("Rotation"=-0.5, "Gyro Angle"=w1785, "Y"=0.0 ("X axis value"), "X"=0.0 ("X axis value"), "RobotDriveDevRef"=w1784) -> ()  [unwired: 4 in, 3 out]
              }
            }
            n680 = Less Or Equal?(x=w1776, y=-80.0) -> (x <= y?=w1775:bool)
          }
        }
        frame #8 {
          n681 = Unbundle By Name(w1791) -> ("SimpleGyroDevRef"=w1790:T3, "RobotDriveDevRef"=w1789:T6)
          n682 = call "WPI_SimpleGyro_Get Angle.vi"("SimpleGyroDevRef"=w1790) -> ("Angle"=w1792:dbl)  [unwired: 8 in, 2 out]
          n683 = call-poly <vilib>:"WPI_RobotDriveHolonomicDrive.vi"("Rotation"=0.0, "Gyro Angle"=w1792, "Y"=0.0, "X"=0.0, "RobotDriveDevRef"=w1789) -> ()  [unwired: 4 in, 3 out]
        }
      }
    }
    frame "Basic", Default {
      n684 = call "WPI_SimpleGyro_RefNum Registry Get.vi"("refnum name"="SimpleGyro") -> ("error out"=w1805:errorcluster, "SimpleGyroDevRef"=w1809:T3)  [unwired: 9 in]
      n685 = call <vilib>:"WPI_RobotDriveRefNum Registry Get.vi"("refnum name"="Four Motors") -> ("error out"=w1804:errorcluster, "RobotDriveDevRef"=w1808:T6)  [unwired: 1 in, 8 out]
      n686 = call <vilib>:"WPI_EncoderRefNum Registry Get.vi"("refnum name"="Left Front Drive Encoder") -> ("error out"=w1803:errorcluster, "EncoderDevRef"=w1807:T15)  [unwired: 9 in]
      n687 = call <vilib>:"WPI_MotorControlRefNum Registry Get.vi"("refnum name"="ARI Motor") -> ("error out"=w1802:errorcluster, "MotorControlDevRef"=w1806:T7)  [unwired: 9 in]
      n688 = call <vilib>:"WPI_RelayRefNum Registry Get.vi"("refnum name"="Clamper Motor") -> ("error out"=w1799:errorcluster, "RelayDevRef"=w1800:T19)  [unwired: 9 in]
      n689 = Bundle("SimpleGyroDevRef"=w1809, "RobotDriveDevRef"=w1808, "EncoderDevRef"=w1807, "MotorControlDevRef"=w1806, "RelayDevRef"=w1800) -> (w1798:T22)  [unwired: 1 in]
      n690 = Bundle("error out"=w1805, "error out"=w1804, "error out"=w1803, "error out"=w1802, "error out"=w1799) -> ()  [unwired: 1 in, 1 out]
      n691 = flat-sequence {
        tunnel: w1798 -> [w1816]
        tunnel: [w1816] -> w1796
        tunnel: [w1822] -> w1815
        tunnel: [w1821] -> w1814
        tunnel: [w1820] -> w1797
        tunnel: w1796 -> [w1819]
        tunnel: w1815 -> [w1852]
        tunnel: w1814 -> [w1851]
        tunnel: w1797 -> [w1847]
        frame #0 {
          n692 = Unbundle By Name(w1816) -> ("SimpleGyroDevRef"=w1818:T3, "EncoderDevRef"=w1817:T15)
          n693 = call "WPI_SimpleGyro_Reset.vi"("SimpleGyroDevRef"=w1818) -> ()  [unwired: 9 in, 2 out]
          n694 = call <vilib>:"WPI_EncoderReset.vi"("EncoderDevRef"=w1817) -> ()  [unwired: 9 in, 2 out]
        }
        frame #1 {
          n695 = while {
            tunnel: [w1833] -> w1822
            tunnel: [w1832] -> w1821
            tunnel: [w1825] -> w1820
            tunnel: w1819 -> [w1824]
            stop <- w1834 stop-if-true
            n696 = Unbundle By Name(w1824) -> ("EncoderDevRef"=w1829:T15, "SimpleGyroDevRef"=w1828:T3, "RobotDriveDevRef"=w1827:T6)
            n697 = Wait (ms)(milliseconds to wait=u32 30) -> ()  [unwired: 1 out]
            n698 = global read "Robot Global Data.vi" "Competition Robot?"() -> (w1831:bool)
            n699 = call "WPI_SimpleGyro_Get Angle.vi"("SimpleGyroDevRef"=w1828) -> ("Angle"=w1823:dbl)  [unwired: 8 in, 2 out]
            n700 = call "Direction Correction.vi"("Gyro Value"=w1823) -> ("Z Value"=w1826:dbl)  [unwired: 10 in]
            n701 = call <vilib>:"WPI_EncoderGet.vi"("EncoderDevRef"=w1829) -> ("error out"=w1832:errorcluster, "Distance"=w1836:dbl, "EncoderDevRef"=w1833:T15)  [unwired: 5 in, 3 out]
            n702 = case shown="False" w1831 {
              tunnel: w1827 -> [w1839 w1843]
              tunnel: w1826 -> [w1838 _]
              tunnel: [w1837 w1842] -> w1825
              frame True {
                n703 = call-poly <vilib>:"WPI_RobotDriveHolonomicDrive.vi"("Rotation"=w1838, "Y"=0.6 ("X axis value"), "X"=0.0 ("X axis value"), "RobotDriveDevRef"=w1839) -> ("RobotDriveDevRef"=w1837:T6)  [unwired: 5 in, 2 out]
              }
              frame False {
                n704 = call-poly <vilib>:"WPI_RobotDriveHolonomicDrive.vi"("Rotation"=0.0, "Y"=-0.4 ("X axis value"), "X"=0.0 ("X axis value"), "RobotDriveDevRef"=w1843) -> ("RobotDriveDevRef"=w1842:T6)  [unwired: 5 in, 2 out]
              }
            }
            n705 = Greater Or Equal?(x=w1836, y=1660.0) -> (x >= y?=w1834:bool)
          }
        }
        frame #2 {
          n706 = while {
            tunnel: w1852 -> [w1855]
            tunnel: w1851 -> [w1854]
            stop <- FALSE stop-if-true
            n707 = call <vilib>:"WPI_EncoderReset.vi"("error in (no error)"=w1854, "EncoderDevRef"=w1855) -> ()  [unwired: 8 in, 2 out]
          }
          n708 = call-poly <vilib>:"WPI_RobotDriveHolonomicDrive.vi"("Rotation"=0.0, "Y"=0.0 ("X axis value"), "X"=0.0 ("X axis value"), "RobotDriveDevRef"=w1847) -> ()  [unwired: 5 in, 3 out]
        }
      }
    }
  }
  n709 = while {
    stop <- FALSE stop-if-true
    n710 = Wait (ms)(milliseconds to wait=u32 20) -> ()  [unwired: 1 out]
    n711 = call <vilib>:"WPI_DriverStationReport Robot Code State.vi"("Autonomous"=TRUE) -> ()  [unwired: 10 in, 1 out]
  }
  n712 = disable-structure shown="Disabled" {
    frame Disabled {
      # "go forward for 1 second"
      # "go forward for 1 second"
      n713 = call <vilib>:"WPI_RobotDriveRefNum Registry Get.vi"("refnum name"="Four Motors") -> ("RobotDriveDevRef"=w1868:T6)  [unwired: 1 in, 9 out]
      n714 = call-poly <vilib>:"WPI_RobotDriveHolonomicDrive.vi"("Rotation"=0.0, "Y"=0.5 ("X axis value"), "X"=0.0 ("X axis value"), "RobotDriveDevRef"=w1868) -> ("Motor Values"=w1865:dbl[], "RobotDriveDevRef"=w1871:T6)  [unwired: 5 in, 1 out]
      n715 = call <vilib>:"WPI_RobotDriveDelayAndUpdateSafety.vi"("Delay (s)"=4.0, "RobotDriveDevRef"=w1871) -> ("RobotDriveDevRef 2"=w1859:T6)  [unwired: 8 in, 1 out]
      n716 = call-poly <vilib>:"WPI_RobotDriveHolonomicDrive.vi"("Rotation"=0.0, "Y"=0.0 ("X axis value"), "X"=0.0 ("X axis value"), "RobotDriveDevRef"=w1859) -> ("Motor Values"=w1860:dbl[])  [unwired: 5 in, 2 out]
      n717 = call-poly <vilib>:"SD Write Value.vi"("Numeric Array"=w1860, "Name"="RobotDrive Motors") -> ()  [unwired: 8 in, 2 out]
      n718 = call-poly <vilib>:"SD Write Value.vi"("Numeric Array"=w1865, "Name"="RobotDrive Motors") -> ()  [unwired: 8 in, 2 out]
    }
    frame Enabled {
    }
  }
